vi "VFP.vi"() -> ()   [LabVIEW 2016]
uses:
  <vilib>/Utility/error.llb/DialogType.ctl
  states/InitializationStates.ctl
  states/DataAcqStates.ctl
  <vilib>/registry/registry.llb/Registry RtKey.ctl
  <vilib>/registry/registry.llb/Registry SAM.ctl
  <vilib>/Utility/error.llb/whitespace.ctl
  <vilib>/Analysis/baseanly.llb/Mean (DBL).vi
  <vilib>/registry/registry.llb/Read Registry Value Simple STR.vi
  Instance           5 11Saved   VFP .vi
  Instance          20 11Saved   VFP .vi
  Instance           6 11Saved   VFP .vi
  Instance          21 11Saved   VFP .vi
  Instance           8 11Saved   VFP .vi
  <vilib>/Analysis/NI_AALPro.lvlib
  <vilib>/Analysis/NI_AALBase.lvlib
panel:
  in  "Clear Graphs":bool
  out "Line of Best Fit":cluster{"type":sgl[], "Best Linear Fit":dbl[]}(graph)
  out "IV Data":cluster{"X":dbl[], "Y":dbl[]}[](graph)
  in  "Save on Start":bool
  out "Rough Resistance (MOhm)":dbl
  out "Done Time":dbl
  out "Current Time":dbl format="%_19f"
  in  "IV_Genfilname":bool
  in  "First Run IV":bool
  out "IV_start":dbl format="%_19f"
  out "Saving":bool
  out "?":path
  out "file or folder exists?":bool
  out "Target Resistance (adjusted Golovochenko)  (MOhm)":dbl
  out "Capillary Diameter (nm)":dbl
  in  "Bare Resistance \n(MOhm)":dbl
  out "Recording IV":bool
  in  "Start/Stop Saving":bool
  in  "Generate Filename":bool
  out "Control Amp Overload":bool caption="CA"
  out "Current Overload":bool caption="I"
  out "Voltage Overload":bool caption="V"
  in  "Legacy Save":bool
  out "Front Panel Window:Title 2":string="Gamry Instruments Virtual Front Panel"
  out "Log File Refnum 2":refnum<file>
  in  "Log File 2":path
  in  "Enable Section":bool
  in  "Desired Pore Size (nm)":dbl
  in  "Membrane Thickness \n(nm)":dbl
  in  "Sealed Resistance\n(MOhm)":dbl
  in  "Solution Conductance":dbl
  in  "Smoothing Parameter":i32=100
  out "Resistance (MOhm)":dbl
  out "Current(nA)":dbl
  in  "Select Graph":u16(ring) items=["V Vs. T, I vs. T", "I vs. V", "V vs. I"]
  out "Family":string
  out "Vf History":sgl[](array[numeric])
  out "Im History":sgl[](array[numeric])
  out "XY Graph Flipped?":bool
  in  "CA Speed":u16(ring)
  in  "I/E Stability":u16(ring)=2 items=["Fast", "Medium Fast", "Normal", "Slow"]
  in  "IchOffsetEnable":bool
  in  "VchOffsetEnable":bool
  in  "Ich Offset":sgl step=0.1 format="%^.3e"
  in  "Vch Offset":sgl step=0.1 format="%^.3e"
  in  "Ich Filter":u16(ring) items=["None", "200 kHz", "1 kHz", "5 Hz"]
  in  "Vch Filter":u16(ring) items=["None", "200 kHz", "1 kHz", "5 Hz"]
  in  "Ich Autorange":bool
  in  "Vch Autorange":bool
  in  "I/E Autorange":bool
  in  "I/E Range":u16(ring)=4 items=["60 pA", "600 pA", "6 nA", "60 nA", "600 nA", "6 µA", "60 µA", "600 µA", "6 mA", "60 mA", "600 mA"]
  in  "Ich Range":u16(ring) items=["30 mV", "300 mV", "3 V"]
  in  "Vch Range":u16(ring) items=["30 mV", "300 mV", "3 V", "12 V"]
  in  "Device":u16(ring) items=["REF600-17061"]
  in  "CtrlMode":u32(ring)=1 items=["Galvanostat", "Potentiostat", "ZRA"]
  in  "Continuous":bool=TRUE
  in  "Acq. Frequency":dbl=100.0 caption="Hz" min=0.001667 max=10000.0 step=1.0 format="%.3f"
  in  "Cycles":u32=1 min=1 step=1
  in  "Signal Type":u16(ring) items=["Take IV Curve"=9, "Sine Wave"=0, "Cosine Wave"=1, "Triangle"=2, "Square Wave"=3, "Sawtooth"=4, "Ramp"=5, "Single Point"=7, "From File"=8]
  in  "Filename":path
  in  "Phase Offset":dbl caption="Degrees" step=1.0 format="%.3f"
  in  "DC Offset":dbl caption="V" step=0.1 format="%^.3e"
  in  "Amplitude":dbl=0.1 caption="V" step=0.1 format="%^.3e"
  in  "Signal Frequency":dbl=1.0 caption="Hz" min=5e-05 max=300000.0 step=0.5 format="%.3f"
  in  "Final":dbl=0.5 caption="V" step=0.1 format="%^.3e"
  in  "Initial":dbl=-0.5 caption="V" step=0.1 format="%^.3e"
  in  "Duty Cycle":dbl=50.0 caption="Percent" min=0.0 max=100.0 step=0.1 format="%.3f"
  in  "Scan Rate":dbl=0.1 caption="V/s" step=0.01 format="%_3f"
  in  "Cell State":bool
  in  "Auto Cell Switch":bool=TRUE
  in  "Start/Stop":bool caption="Start"
  out "Confirm Exit?":bool
  out "?":sgl[][](graph)
  out "I vs. V":cluster{dbl, dbl}[](graph)
  out "SetCell":bool
  out "Cell Val Change NewVal":bool
  out "Version":string
  in  "[user-defined codes]":u32[](array[numeric])=[3758096430]
  in  "[user-defined descriptions]":string[](array[string])=["Device Not Authorized"]
  out "Taking Data":bool
  out "Front Panel Window:Title":string="Gamry Instruments Virtual Front Panel"
  in  "Log File":path
  out "Device Gone":bool
  out "Index of Device (Device Change)":i32
  out "milliseconds to wait":u32=150
  in  "Close":bool
  out "From File Refnum":refnum<file>
  out "Data Handlers":T1
  out "Log File Refnum":refnum<file>
  out "ForcePstatFunctionUpdate":bool
  out "File Data":string
  out "Device List Change Callback":refnum<k27>
  in  "Device List Change":bool
  out "Device Open":bool
  out "Section":string
  in  "GAMRYCOMLib.IGamrySignalArray":refnum<k7>
  in  "GAMRYCOMLib.IGamryDtaqIv":refnum<k7>
  in  "GAMRYCOMLib.IGamryPstat":refnum<k7>
  in  "GAMRYCOMLib.IGamryDeviceList":refnum<k7>
  out "DataDone Callback":refnum<k27>
  out "DataDone?":bool
  out "Dtaq Graph Callback":refnum<k27>
  in  "GAMRYCOMLib.IGamrySignal":refnum<k7>
  out "Signal":refnum<k7>
  out "Dtaq":refnum<k7>
  out "Pstat":refnum<k7>
  out "Device List":refnum<k7>
  out "First I/E Range":i32
  out "Section List":string[](array[string])=["PC5600-00002"]
  # "amoureux"
  # "Overloads"
  # "Save"
  # "Live View"
  # "1"
  # "2"
  # "displacing carbon atoms since 2018"
  # "Signal Generation"
  # "Nanopore Creator"
  # "Device Settings"
  # "Experiment Control"
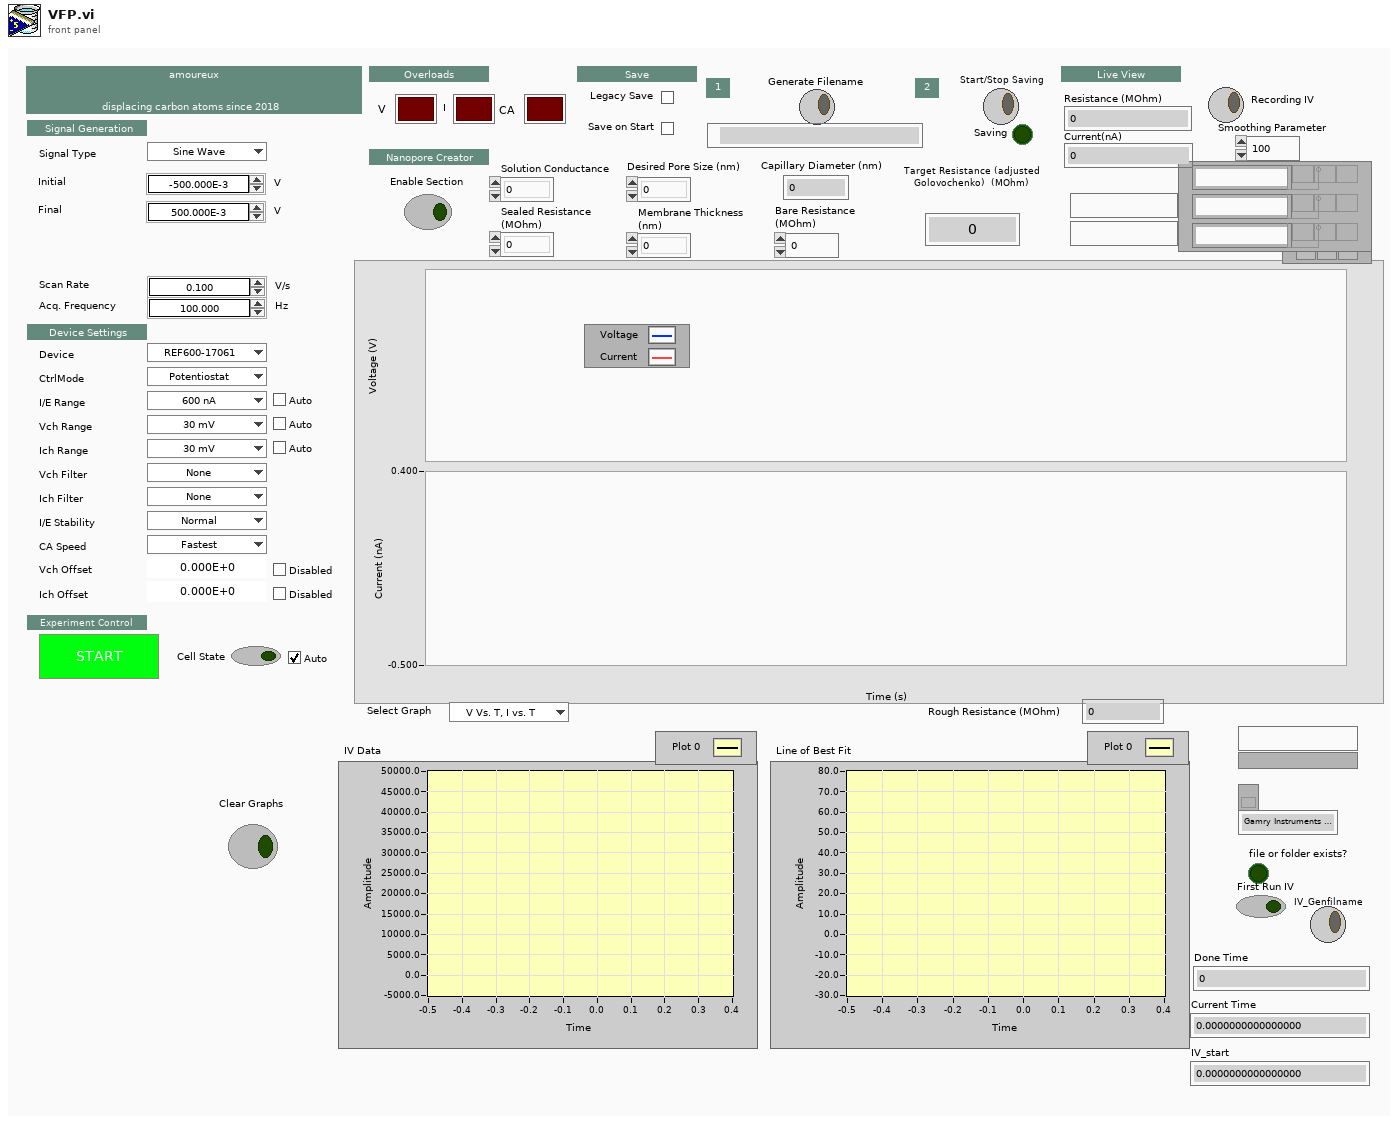
[diagram p1: front panel]
types:
  T1 = cluster{"Vs. T":refnum<vi>, "I vs. V":refnum<vi>, "Log File Refnum":refnum<vi>}
  T2 = typedef "InitializationStates.ctl" = enum16{"Initialize COM", "Load Device List", "Load Range Strings", "Setup Ranges", "Adjust Menu", "STOP"}
  T3 = typedef "DataAcqStates.ctl" = enum16{"Initialize", "Initialize Objects", "Generate Signal", "Data Acq Setup", "Acquire Data", "Cleanup", "STOP"}
  T4 = typedef "Registry SAM.ctl" = enum32{"KEY_QUERY_VALUE", "KEY_SET_VALUE", "KEY_CREATE_SUB_KEY", "KEY_ENUMERATE_SUB_KEYS", "KEY_NOTIFY", "KEY_CREATE_LINK", "KEY_READ", "KEY_WRITE", "KEY_ALL_ACCESS", "KEY_READ | KEY_WRITE"}
  T5 = typedef "Registry RtKey.ctl" = enum32{"HKEY_CLASSES_ROOT", "HKEY_CURRENT_USER", "HKEY_LOCAL_MACHINE", "HKEY_USERS", "HKEY_PERFORMANCE_DATA", "HKEY_CURRENT_CONFIG", "HKEY_DYN_DATA"}
  T6 = enum16{"open", "open or create", "create or replace", "create", "open (read only)"}
  T7 = cluster{"Ctrl Reference":refnum<vi>, "I vs. V":refnum<vi>, "Log File Refnum":refnum<vi>}
  T8 = cluster{"I/E Ranges":string[], "First I/E Range":i32, "VchRanges":string[], "IchRanges":string[], "AchRanges":string[], "VchFilters":string[], "IchFilters":string[], "AchFilters":string[], "Family":string, "CA Speeds":string[]}
  T9 = enum32{"existing file", "new file", "new or existing file", "existing dir", "new dir", "new or existing dir", "existing file (use LLBs)", "new file (use LLBs)", "new or existing file (use LLBs)", "new or existing file or directory (use LLBs)"}
  T10 = typedef "Registry refnum.ctl" = refnum<k1>
  T11 = typedef "whitespace.ctl" = u16
  T12 = cluster{"I Overload":bool, "CA Overload":bool, "V Overload":bool, "I ADC Railed":bool, "V ADC Railed":bool}
  T13 = enum32{"invalid app kind", "Development System", "Run Time System", "Student Edition", "Embedded LabVIEW", "Evaluation", "Custom"}
  T14 = typedef "DialogType.ctl" = u16
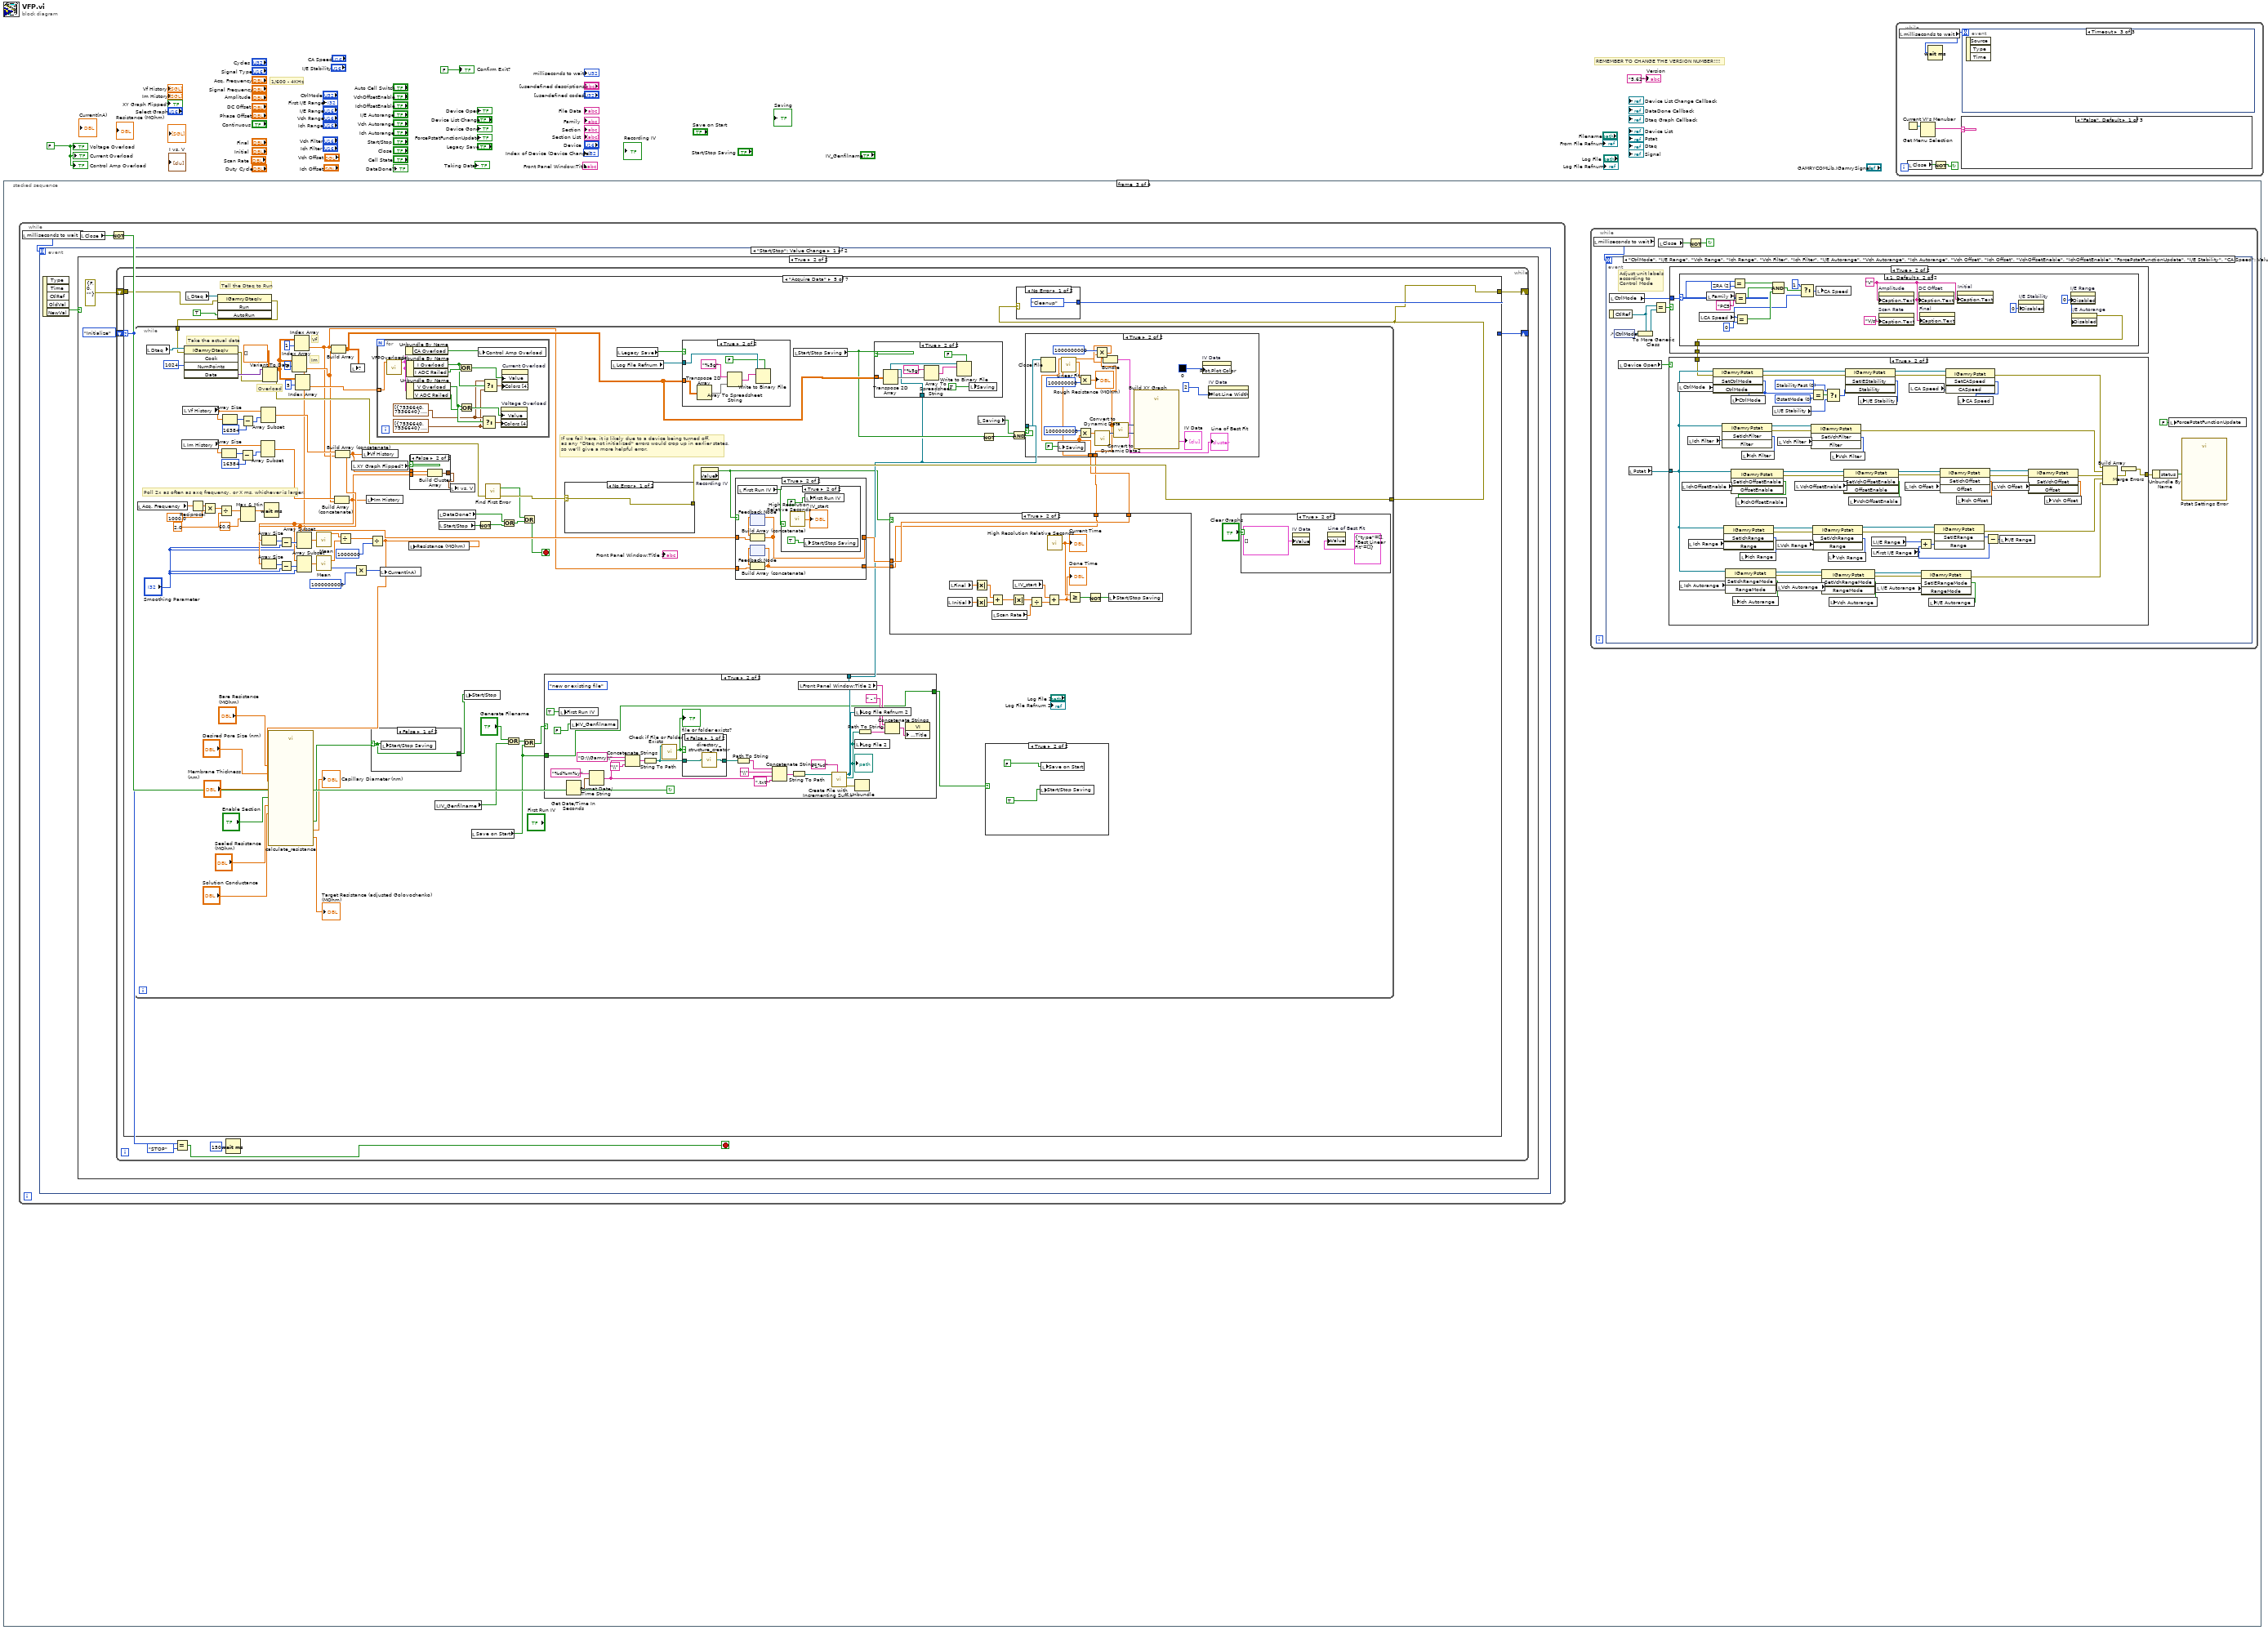
[diagram p0: block diagram]
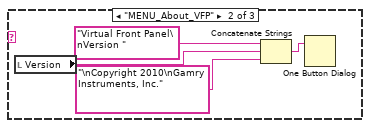
[diagram p2: hidden frame]
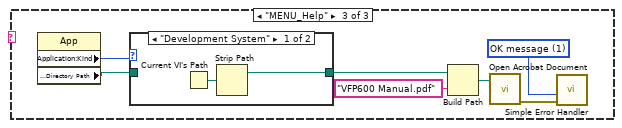
[diagram p3: hidden frame]
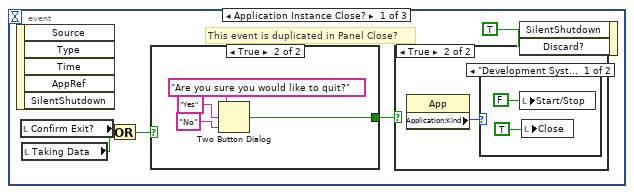
[diagram p5: hidden frame]
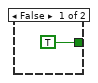
[diagram p6: hidden frame]
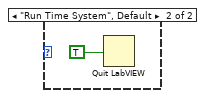
[diagram p8: hidden frame]
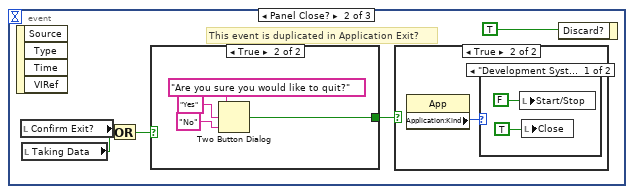
[diagram p9: hidden frame]
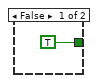
[diagram p10: hidden frame]
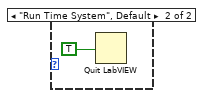
[diagram p12: hidden frame]
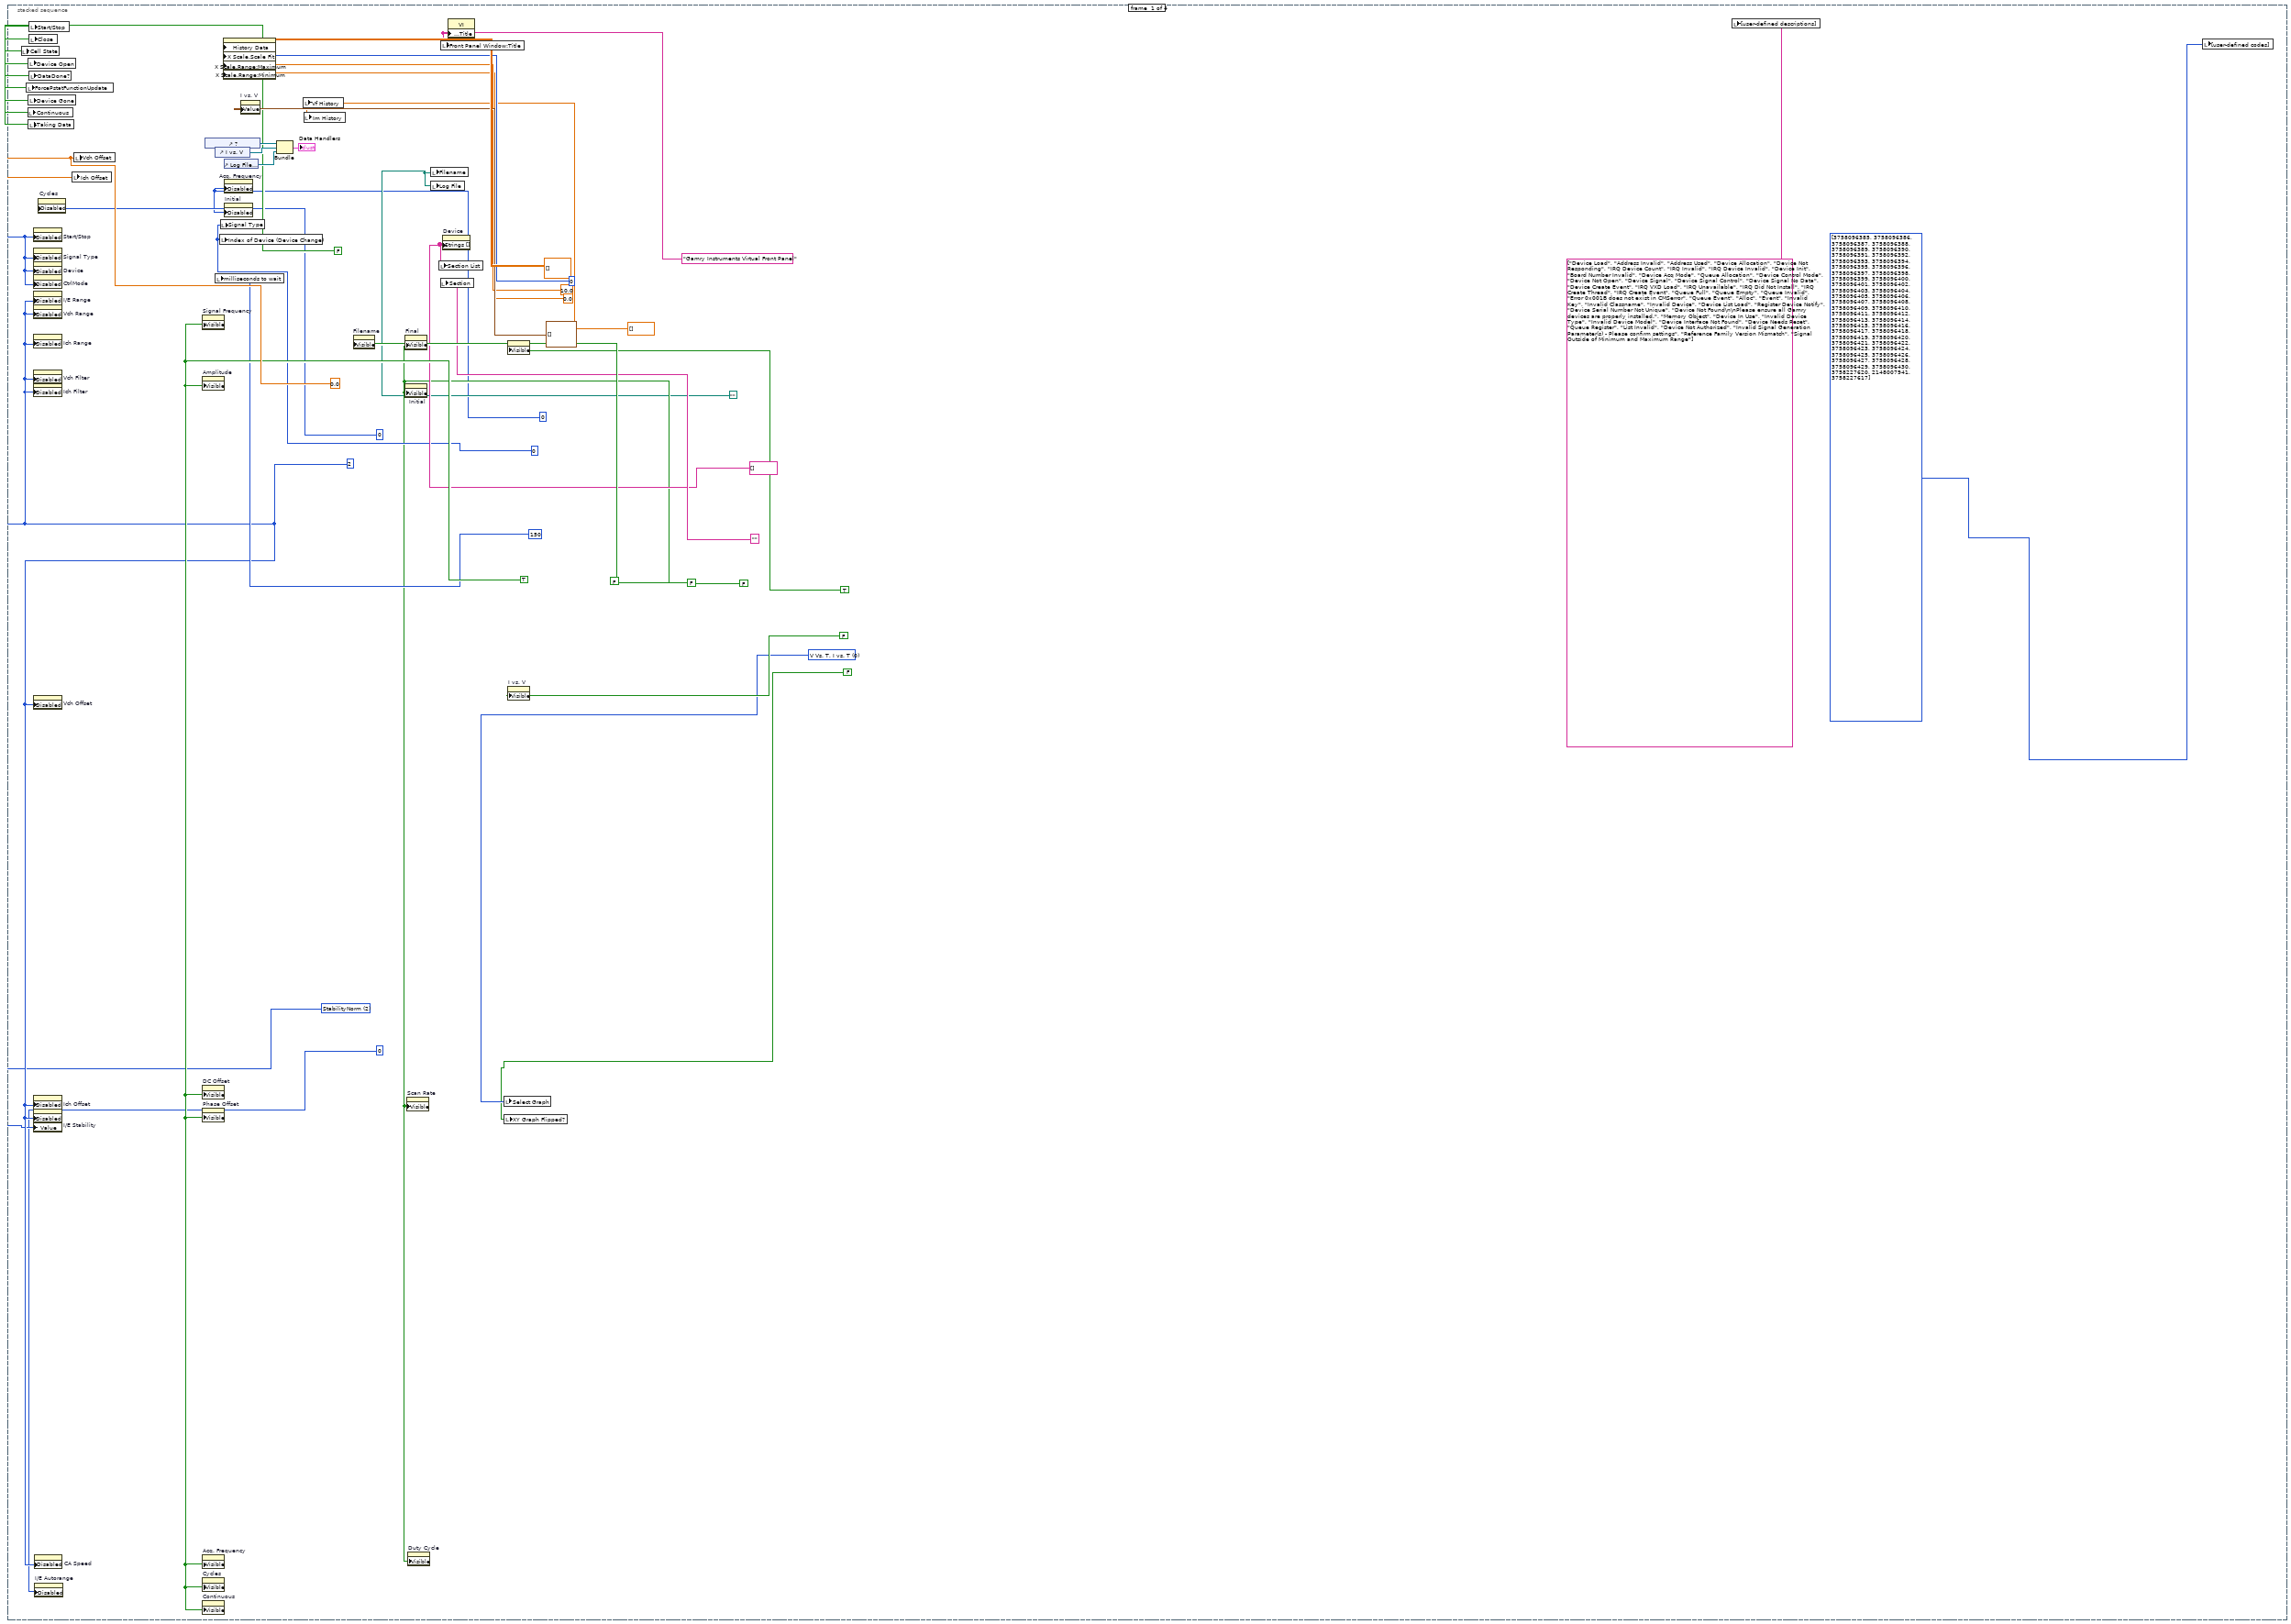
[diagram p13: hidden frame]
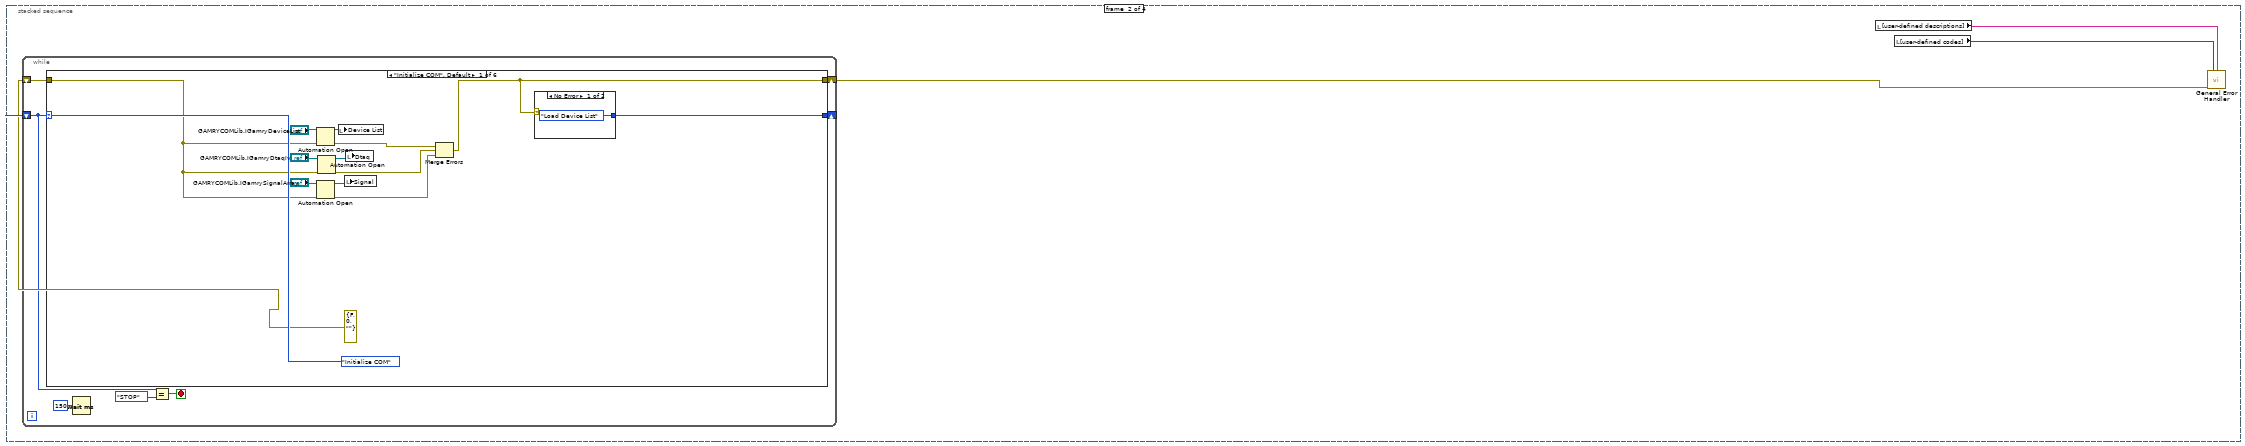
[diagram p14: hidden frame]
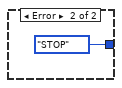
[diagram p15: hidden frame]
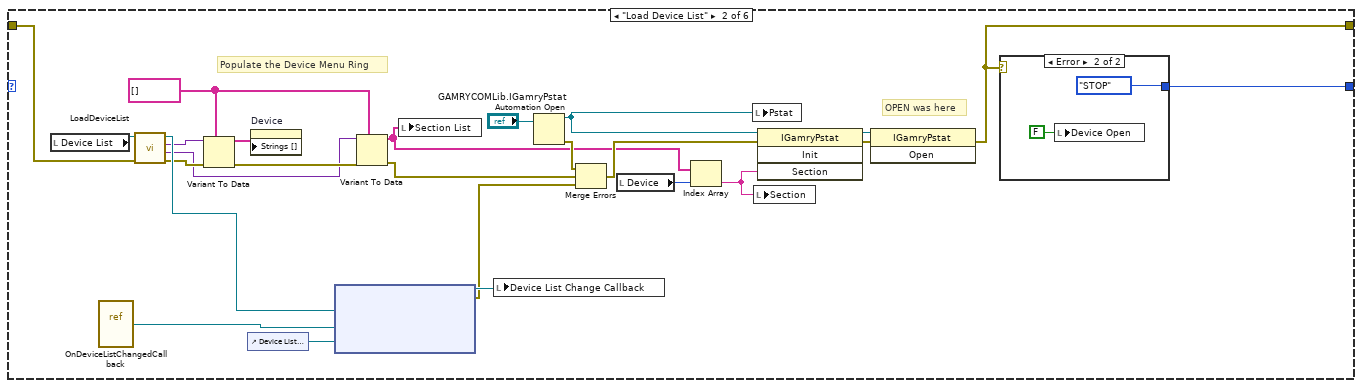
[diagram p16: hidden frame]
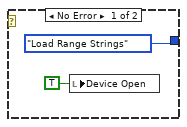
[diagram p17: hidden frame]
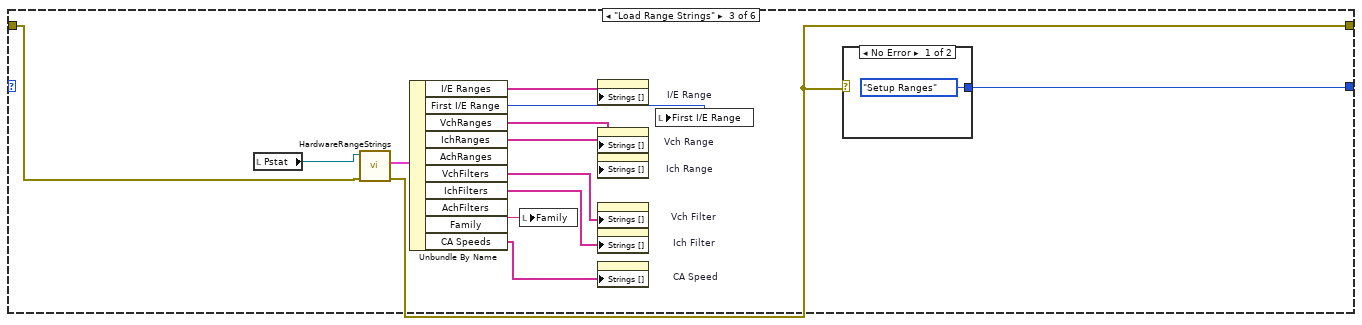
[diagram p18: hidden frame]
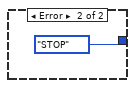
[diagram p19: hidden frame]
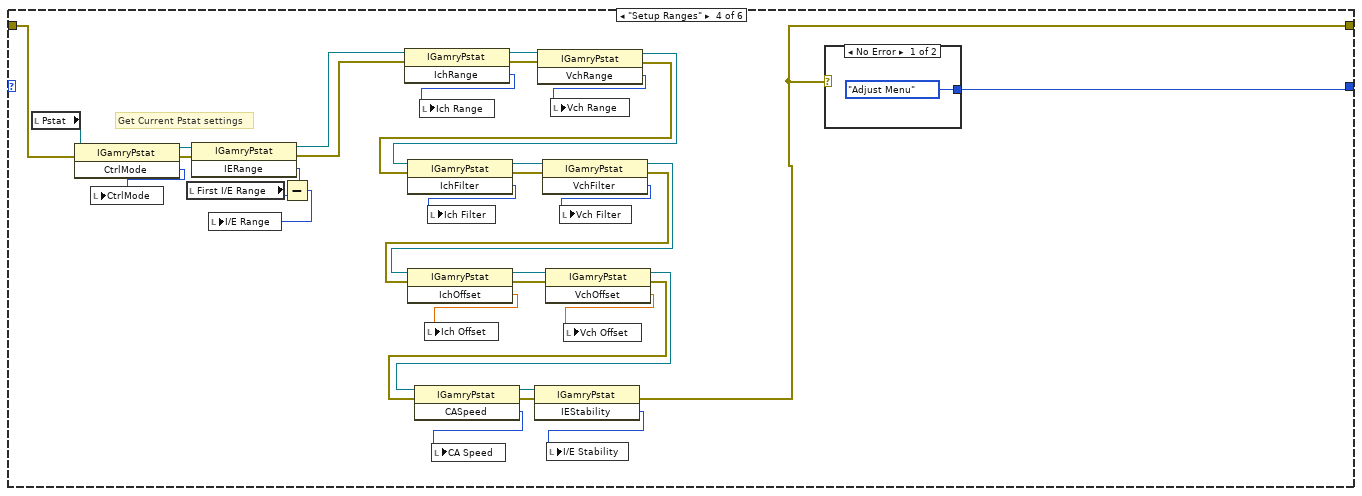
[diagram p20: hidden frame]
diagram:
  w1 = FALSE
  # "REMEMBER TO CHANGE THE VERSION NUMBER!!!!"
  # "1/600 - 4KHz"
  n1 = stacked-sequence {
    frame #0 {
      w5 = sgl[] [] ("Vf History")
      w7 = u16 0 items=["V Vs. T, I vs. T", "I vs. V", "V vs. I"] ("Select Graph")
      w12 = path ""
      w13 = 2 items=["StabilityFast", "StabilityMedFast", "StabilityNorm", "StabilitySlow"] ("Stability")
      w20 = "Gamry Instruments Virtual Front Panel" ("Front Panel Window:Title")
      w15 = FALSE ("Visible")
      w8 = u8 0 ("Disabled")
      w14 = u8 2 ("Disabled")
      (unwired) FALSE ("Visible")
      w30 = TRUE ("Visible")
      w34 = sgl 0.0 ("Vch Offset")
      w19 = FALSE ("I/E Autorange 2")
      w24 = u32 0 ("Zero")
      w25 = string[] [] ("Strings []")
      n2 = local write "Cell State"(w19) -> ()
      n3 = local write "ForcePstatFunctionUpdate"(w19) -> ()
      n4 = local write "Continuous"(w19) -> ()
      n5 = local write "Device Open"(w19) -> ()
      n6 = local write "Device Gone"(w19) -> ()
      n7 = local write "Taking Data"(w19) -> ()
      n8 = local write "DataDone?"(w19) -> ()
      n9 = local write "Start/Stop"(w19) -> ()
      n10 = local write "Close"(w19) -> ()
      n11 = property on="Start/Stop" class="Bool (strict)"("Disabled"=w14) -> ()  [unwired: 2 in, 2 out]
      n12 = property on="Signal Type" class="Ring (strict)"("Disabled"=w14) -> ()  [unwired: 2 in, 2 out]
      n13 = property on="Device" class="Ring (strict)"("Disabled"=w14) -> ()  [unwired: 2 in, 2 out]
      n14 = property on="CtrlMode" class="Ring (strict)"("Disabled"=w14) -> ()  [unwired: 2 in, 2 out]
      n15 = property on="I/E Range" class="Ring (strict)"("Disabled"=w14) -> ()  [unwired: 2 in, 2 out]
      n16 = property on="Vch Range" class="Ring (strict)"("Disabled"=w14) -> ()  [unwired: 2 in, 2 out]
      n17 = property on="Ich Range" class="Ring (strict)"("Disabled"=w14) -> ()  [unwired: 2 in, 2 out]
      n18 = property on="Vch Filter" class="Ring (strict)"("Disabled"=w14) -> ()  [unwired: 2 in, 2 out]
      n19 = property on="Ich Filter" class="Ring (strict)"("Disabled"=w14) -> ()  [unwired: 2 in, 2 out]
      n20 = property on="Vch Offset" class="DigNum (strict)"("Disabled"=w14) -> ()  [unwired: 2 in, 2 out]
      n21 = property on="Ich Offset" class="DigNum (strict)"("Disabled"=w14) -> ()  [unwired: 2 in, 2 out]
      n22 = property on="I/E Stability" class="Ring (strict)"("Disabled"=w14, "Value"=w13) -> ()  [unwired: 2 in, 2 out]
      n23 = property on="CA Speed" class="Ring (strict)"("Disabled"=w14) -> ()  [unwired: 2 in, 2 out]
      n24 = property on="I/E Autorange" class="Bool (strict)"("Disabled"=u8 0) -> ()  [unwired: 2 in, 2 out]
      n25 = property on="Cycles" class="DigNum (strict)"("Disabled"=0) -> ()  [unwired: 2 in, 2 out]
      n26 = local write "Ich Offset"(w34) -> ()
      n27 = local write "Vch Offset"(w34) -> ()
      n28 = property on="Signal Frequency" class="DigNum (strict)"("Visible"=w30) -> ()  [unwired: 2 in, 2 out]
      n29 = property on="Amplitude" class="DigNum (strict)"("Visible"=w30) -> ()  [unwired: 2 in, 2 out]
      n30 = property on="DC Offset" class="DigNum (strict)"("Visible"=w30) -> ()  [unwired: 2 in, 2 out]
      n31 = property on="Phase Offset" class="DigNum (strict)"("Visible"=w30) -> ()  [unwired: 2 in, 2 out]
      n32 = property on="Acq. Frequency" class="DigNum (strict)"("Visible"=w30) -> ()  [unwired: 2 in, 2 out]
      n33 = property on="Cycles" class="DigNum (strict)"("Visible"=w30) -> ()  [unwired: 2 in, 2 out]
      n34 = property on="Continuous" class="Bool (strict)"("Visible"=w30) -> ()  [unwired: 2 in, 2 out]
      n35 = control-ref of="?"() -> (w33:refnum<vi>)
      n36 = control-ref of="I vs. V"() -> (w32:refnum<vi>)
      n37 = local write "milliseconds to wait"(u32 150 ("milliseconds to wait")) -> ()
      n38 = local write "Index of Device (Device Change)"(w24) -> ()
      n39 = local write "Signal Type"(w24) -> ()
      n40 = property class="WFChart (strict)"("History Data"=sgl[][] [], "X Scale.Scale Fit"=u8 0, "X Scale.Range:Maximum"=10.0, "X Scale.Range:Minimum"=0.0) -> ()  [unwired: 2 in, 2 out]
      n41 = control-ref of="Log File Refnum"() -> (w28:refnum<vi>)
      n42 = property on="Acq. Frequency" class="DigNum (strict)"("Disabled"=w8) -> ()  [unwired: 2 in, 2 out]
      n43 = property on="Initial" class="DigNum (strict)"("Disabled"=w8) -> ()  [unwired: 2 in, 2 out]
      n44 = property on="I vs. V" class="XYGraph (strict)"("Value"=cluster{dbl, dbl}[] [] ("I vs. V")) -> ()  [unwired: 2 in, 2 out]
      n45 = Bundle("Ctrl Reference"=w33, "I vs. V"=w32, "Log File Refnum"=w28) -> (→"Data Handlers":T7)  [unwired: 1 in]
      n46 = local write "Vf History"(w5) -> ()
      n47 = local write "Im History"(w5) -> ()
      n48 = property on="Filename" class="Path"("Visible"=FALSE) -> ()  [unwired: 2 in, 2 out]
      n49 = property on="Final" class="DigNum (strict)"("Visible"=w15) -> ()  [unwired: 2 in, 2 out]
      n50 = property on="Initial" class="DigNum (strict)"("Visible"=w15) -> ()  [unwired: 2 in, 2 out]
      n51 = property on="Scan Rate" class="DigNum (strict)"("Visible"=w15) -> ()  [unwired: 2 in, 2 out]
      n52 = property on="Duty Cycle" class="DigNum (strict)"("Visible"=w15) -> ()  [unwired: 2 in, 2 out]
      n53 = local write "Filename"(w12) -> ()
      n54 = local write "Log File"(w12) -> ()
      n55 = local write "Section List"(w25) -> ()
      n56 = local write "Section"("" ("Section")) -> ()
      n57 = local write "Front Panel Window:Title"(w20) -> ()
      n58 = property on="Device" class="Ring (strict)"("Strings []"=w25) -> ()  [unwired: 2 in, 2 out]
      n59 = property class="VI"("Front Panel Window:Title"=w20) -> ()  [unwired: 2 in, 2 out]
      n60 = local write "Select Graph"(w7) -> ()
      n61 = local write "XY Graph Flipped?"(FALSE ("XY Graph Flipped?")) -> ()
      n62 = property class="WFChart (strict)"("Visible"=TRUE) -> ()  [unwired: 2 in, 2 out]
      n63 = property on="I vs. V" class="XYGraph (strict)"("Visible"=FALSE) -> ()  [unwired: 2 in, 2 out]
      n64 = local write "[user-defined descriptions]"(string[] ["Device Load", "Address Invalid", "Address Used", "Device Allocation", "Device Not Responding", "IRQ Device Count", "IRQ Invalid", "IRQ Device Invalid", "Device Init", "Board Number Invalid", "Device Acq Mode", "Queue Allocation", "Device Control Mode", "Device Not Open", "Device Signal", "Device Signal Control", "Device Signal No Data", "Device Create Event", "IRQ VXD Load", "IRQ Unavailable", "IRQ Did Not Install", "IRQ Create Thread", "IRQ Create Event", "Queue Full", "Queue Empty", "Queue Invalid", "Error 0x001B does not exist in CMSerror", "Queue Event", "Alloc", "Event", "Invalid Key", "Invalid Classname", "Invalid Device", "Device List Load", "Register Device Notify", "Device Serial Number Not Unique", "Device Not Found\n\nPlease ensure all Gamry devices are properly installed.", "Memory Object", "Device In Use", "Invalid Device Type", "Invalid Device Model", "Device Interface Not Found", "Device Needs Reset", "Queue Register", "List Invalid", "Device Not Authorized", "Invalid Signal Generation Parameter(s) - Please confirm settings", "Reference Family Version Mismatch", "Signal Outside of Minimum and Maximum Range"] ("[user-defined descriptions]")) -> ()
      n65 = local write "[user-defined codes]"(u32[] [3758096385, 3758096386, 3758096387, 3758096388, 3758096389, 3758096390, 3758096391, 3758096392, 3758096393, 3758096394, 3758096395, 3758096396, 3758096397, 3758096398, 3758096399, 3758096400, 3758096401, 3758096402, 3758096403, 3758096404, 3758096405, 3758096406, 3758096407, 3758096408, 3758096409, 3758096410, 3758096411, 3758096412, 3758096413, 3758096414, 3758096415, 3758096416, 3758096417, 3758096418, 3758096419, 3758096420, 3758096421, 3758096422, 3758096423, 3758096424, 3758096425, 3758096426, 3758096427, 3758096428, 3758096429, 3758096430, 3758227620, 2148007941, 3758227617] ("[user-defined codes]")) -> ()
    }
    frame #1 {
      n66 = while {
        shift-right: [w41] -> _
        shift-left: InitializationStates."Initialize COM" ("Initialization States") -> [w47]
        shift-right: [w43] -> w36
        shift-left: errorcluster {"status"=FALSE, "code"=0, "source"=""} ("error out") -> [w42]
        stop <- w45 stop-if-true
        n67 = case shown="\"Initialize COM\", Default" w47 {
          tunnel: [w49 w62 w91 w106 w142 w161] -> w43
          tunnel: w42 -> [w50 w67 w93 w133 w143 w161]
          tunnel: [w48 w65 w97 w132 w151 InitializationStates."STOP" ("Initialization States")] -> w41
          frame "Initialize COM", Default {
            n68 = Automation Open(error in (no error)=w50, Automation Refnum="GAMRYCOMLib.IGamryDeviceList") -> (Automation Refnum=w59:refnum<k7>, error out=w56:errorcluster)  [unwired: 2 in]
            n69 = Automation Open(error in (no error)=w50, Automation Refnum="GAMRYCOMLib.IGamrySignalArray") -> (Automation Refnum=w52:refnum<k7>, error out=w58:errorcluster)  [unwired: 2 in]
            n70 = Automation Open(error in (no error)=w50, Automation Refnum="GAMRYCOMLib.IGamryDtaqIv") -> (Automation Refnum=w51:refnum<k7>, error out=w57:errorcluster)  [unwired: 2 in]
            n71 = local write "Device List"(w59) -> ()
            n72 = local write "Signal"(w52) -> ()
            n73 = local write "Dtaq"(w51) -> ()
            n74 = Merge Errors(w56, w57, w58) -> (w49:errorcluster)
            n75 = case shown="No Error" w49 {
              tunnel: [InitializationStates."Load Device List" ("Initialization States") InitializationStates."STOP" ("Initialization States")] -> w48
              frame No Error {
              }
              frame Error {
              }
            }
          }
          frame "Load Device List" {
            w69 = string[] []
            # "OPEN was here"
            # "Populate the Device Menu Ring"
            n76 = local read "Device List"() -> (w86:refnum<k7>)
            n77 = vi-ref "OnDeviceListChangedCallback.vi"() -> ("vi reference"=w75:refnum<vi>)
            n78 = call "LoadDeviceList.vi"("Error In"=w67, "GAMRYCOMLib.IGamryDeviceList In"=w86) -> ("Error Out"=w82:errorcluster, "EnumSections"=w81:variant, "EnumLabels"=w80:variant, "GAMRYCOMLib.IGamryDeviceList Out"=w85:refnum<k7>)  [unwired: 4 in]
            n79 = Variant To Data(error in=w82, type=w69, Variant=w80) -> (data=w68:string[], error out=w84:errorcluster)
            n80 = control-ref of="Device List Change"() -> (w74:refnum<vi>)
            n81 = property on="Device" class="Ring (strict)"("Strings []"=w68) -> ()  [unwired: 2 in, 2 out]
            n82 = node(w85, w75, w74) -> (w76:refnum<k27>, w66:errorcluster)  [unwired: 2 in]
            n83 = Variant To Data(error in=w84, type=w69, Variant=w81) -> (data=w77:string[], error out=w83:errorcluster)
            n84 = local write "Section List"(w77) -> ()
            n85 = local write "Device List Change Callback"(w76) -> ()
            n86 = Automation Open(Automation Refnum="GAMRYCOMLib.IGamryPstat") -> (Automation Refnum=w73:refnum<k7>, error out=w78:errorcluster)  [unwired: 3 in]
            n87 = Merge Errors(w78, w83, w66) -> (w79:errorcluster)
            n88 = local read "Device"() -> (w71:u16)
            n89 = Index Array(array=w77, index=w71) -> (element=w72:string)
            n90 = local write "Pstat"(w73) -> ()
            n91 = local write "Section"(w72) -> ()
            n92 = invoke class="IGamryPstat" method="Init"(reference=w73, error in=w79, "Section"=w72) -> (reference out=w63:refnum<k7>, error out=w64:errorcluster)  [unwired: 1 in, 2 out]
            n93 = invoke class="IGamryPstat" method="Open"(reference=w63, error in=w64) -> (error out=w62:errorcluster)  [unwired: 1 in, 2 out]
            n94 = case shown="Error" w62 {
              tunnel: [InitializationStates."Load Range Strings" ("Initialization States") InitializationStates."STOP" ("Initialization States")] -> w65
              frame No Error {
                n95 = local write "Device Open"(TRUE ("Device Open")) -> ()
              }
              frame Error {
                n96 = local write "Device Open"(FALSE ("Device Open")) -> ()
              }
            }
          }
          frame "Load Range Strings" {
            n97 = local read "Pstat"() -> (w94:refnum<k7>)
            n98 = call "HardwareRangeStrings.vi"("error in (no error)"=w93, "Pstat IN"=w94) -> ("error out"=w91:errorcluster, "Hardware Strings"=w92:T8)  [unwired: 7 in, 1 out]
            n99 = Unbundle By Name(w92) -> ("I/E Ranges"=w101:string[], "First I/E Range"=w98:i32, "VchRanges"=w99:string[], "IchRanges"=w100:string[], "VchFilters"=w102:string[], "IchFilters"=w103:string[], "Family"=w95:string, "CA Speeds"=w96:string[])  [unwired: 2 out]
            n100 = local write "Family"(w95) -> ()
            n101 = property on="I/E Range" class="Ring (strict)"("Strings []"=w101) -> ()  [unwired: 2 in, 2 out]
            n102 = property on="Vch Range" class="Ring (strict)"("Strings []"=w99) -> ()  [unwired: 2 in, 2 out]
            n103 = property on="Ich Range" class="Ring (strict)"("Strings []"=w100) -> ()  [unwired: 2 in, 2 out]
            n104 = property on="Vch Filter" class="Ring (strict)"("Strings []"=w102) -> ()  [unwired: 2 in, 2 out]
            n105 = property on="Ich Filter" class="Ring (strict)"("Strings []"=w103) -> ()  [unwired: 2 in, 2 out]
            n106 = property on="CA Speed" class="Ring (strict)"("Strings []"=w96) -> ()  [unwired: 2 in, 2 out]
            n107 = local write "First I/E Range"(w98) -> ()
            n108 = case shown="No Error" w91 {
              tunnel: [InitializationStates."Setup Ranges" ("Initialization States") InitializationStates."STOP" ("Initialization States")] -> w97
              frame No Error {
              }
              frame Error {
              }
            }
          }
          frame "Setup Ranges" {
            # "Get Current Pstat settings"
            n109 = local read "Pstat"() -> (w134:refnum<k7>)
            n110 = invoke class="IGamryPstat" method="CtrlMode"(reference=w134, error in=w133) -> (reference out=w138:refnum<k7>, error out=w139:errorcluster, "CtrlMode"=w136:i32)  [unwired: 1 in]
            n111 = local write "CtrlMode"(w136) -> ()
            n112 = local read "First I/E Range"() -> (w131:i32)
            n113 = invoke class="IGamryPstat" method="IERange"(reference=w138, error in=w139) -> (reference out=w108:refnum<k7>, error out=w107:errorcluster, "IERange"=w135:i32)  [unwired: 1 in]
            n114 = Subtract(x=w135, y=w131) -> (x-y=w137:i32)
            n115 = local write "I/E Range"(w137) -> ()
            n116 = invoke class="IGamryPstat" method="IchRange"(reference=w108, error in=w107) -> (reference out=w113:refnum<k7>, error out=w112:errorcluster, "IchRange"=w110:i32)  [unwired: 1 in]
            n117 = local write "Ich Range"(w110) -> ()
            n118 = invoke class="IGamryPstat" method="VchRange"(reference=w113, error in=w112) -> (reference out=w126:refnum<k7>, error out=w109:errorcluster, "VchRange"=w111:i32)  [unwired: 1 in]
            n119 = invoke class="IGamryPstat" method="IchFilter"(reference=w126, error in=w109) -> (reference out=w121:refnum<k7>, error out=w120:errorcluster, "IchFilter"=w122:i32)  [unwired: 1 in]
            n120 = local write "Ich Filter"(w122) -> ()
            n121 = invoke class="IGamryPstat" method="VchFilter"(reference=w121, error in=w120) -> (reference out=w128:refnum<k7>, error out=w127:errorcluster, "VchFilter"=w123:i32)  [unwired: 1 in]
            n122 = invoke class="IGamryPstat" method="IchOffset"(reference=w128, error in=w127) -> (reference out=w118:refnum<k7>, error out=w119:errorcluster, "IchOffset"=w124:sgl)  [unwired: 1 in]
            n123 = local write "Ich Offset"(w124) -> ()
            n124 = invoke class="IGamryPstat" method="VchOffset"(reference=w118, error in=w119) -> (reference out=w130:refnum<k7>, error out=w129:errorcluster, "VchOffset"=w125:sgl)  [unwired: 1 in]
            n125 = invoke class="IGamryPstat" method="CASpeed"(reference=w130, error in=w129) -> (reference out=w114:refnum<k7>, error out=w115:errorcluster, "CASpeed"=w117:i32)  [unwired: 1 in]
            n126 = local write "CA Speed"(w117) -> ()
            n127 = invoke class="IGamryPstat" method="IEStability"(reference=w114, error in=w115) -> (error out=w106:errorcluster, "IEStability"=w116:i32)  [unwired: 1 in, 1 out]
            n128 = local write "I/E Stability"(w116) -> ()
            n129 = local write "Vch Range"(w111) -> ()
            n130 = local write "Vch Filter"(w123) -> ()
            n131 = local write "Vch Offset"(w125) -> ()
            n132 = case shown="No Error" w106 {
              tunnel: [InitializationStates."Adjust Menu" ("Initialization States") InitializationStates."STOP" ("Initialization States")] -> w132
              frame No Error {
              }
              frame Error {
              }
            }
          }
          frame "Adjust Menu" {
            n133 = local read "CtrlMode"() -> (w150:u32)
            n134 = case shown="0" w150 {
              tunnel: ["V" ("Caption.Text") "A" ("Caption.Text")] -> w149
              tunnel: ["V/s" ("Caption.Text") "A/s" ("Caption.Text")] -> w148
              frame 1, Default {
              }
              frame 0 {
              }
            }
            n135 = property on="Amplitude" class="DigNum (strict)"(error in=w143, "Caption.Text"=w149) -> (error out=w147:errorcluster)  [unwired: 1 in, 1 out]
            n136 = property on="DC Offset" class="DigNum (strict)"(error in=w147, "Caption.Text"=w149) -> (error out=w146:errorcluster)  [unwired: 1 in, 1 out]
            n137 = property on="Initial" class="DigNum (strict)"(error in=w146, "Caption.Text"=w149) -> (error out=w145:errorcluster)  [unwired: 1 in, 1 out]
            n138 = property on="Final" class="DigNum (strict)"(error in=w145, "Caption.Text"=w149) -> (error out=w144:errorcluster)  [unwired: 1 in, 1 out]
            n139 = property on="Scan Rate" class="DigNum (strict)"(error in=w144, "Caption.Text"=w148) -> (error out=w142:errorcluster)  [unwired: 1 in, 1 out]
            n140 = case shown="Error" w142 {
              tunnel: [InitializationStates."STOP" ("Initialization States") InitializationStates."STOP" ("Initialization States")] -> w151
              frame No Error {
                w156 = u8 0 ("Disabled")
                # "Enable appropriate menu stuff"
                n141 = property on="Start/Stop" class="Bool (strict)"("Disabled"=w156) -> ()  [unwired: 2 in, 2 out]
                n142 = property on="Device" class="Ring (strict)"("Disabled"=w156) -> ()  [unwired: 2 in, 2 out]
                n143 = property on="CtrlMode" class="Ring (strict)"("Disabled"=w156) -> ()  [unwired: 2 in, 2 out]
                n144 = property on="Signal Type" class="Ring (strict)"("Disabled"=w156) -> ()  [unwired: 2 in, 2 out]
                n145 = property on="I/E Range" class="Ring (strict)"("Disabled"=w156) -> ()  [unwired: 2 in, 2 out]
                n146 = property on="Vch Range" class="Ring (strict)"("Disabled"=w156) -> ()  [unwired: 2 in, 2 out]
                n147 = property on="Ich Range" class="Ring (strict)"("Disabled"=w156) -> ()  [unwired: 2 in, 2 out]
                n148 = property on="Vch Filter" class="Ring (strict)"("Disabled"=w156) -> ()  [unwired: 2 in, 2 out]
                n149 = property on="Ich Filter" class="Ring (strict)"("Disabled"=w156) -> ()  [unwired: 2 in, 2 out]
                n150 = property on="Vch Offset" class="DigNum (strict)"("Disabled"=w156) -> ()  [unwired: 2 in, 2 out]
                n151 = property on="Ich Offset" class="DigNum (strict)"("Disabled"=w156) -> ()  [unwired: 2 in, 2 out]
                n152 = property on="I/E Stability" class="Ring (strict)"("Disabled"=w156) -> ()  [unwired: 2 in, 2 out]
                n153 = property on="CA Speed" class="Ring (strict)"("Disabled"=w156) -> ()  [unwired: 2 in, 2 out]
              }
              frame Error {
                w160 = u16 0 items=[""] ("Device")
                w158 = u8 2 ("Disabled")
                # "Disable appropriate menu stuff"
                n154 = property on="Start/Stop" class="Bool (strict)"("Disabled"=w158) -> ()  [unwired: 2 in, 2 out]
                n155 = property on="CtrlMode" class="Ring (strict)"("Disabled"=w158) -> ()  [unwired: 2 in, 2 out]
                n156 = property on="Device" class="Ring (strict)"("Disabled"=w158, "Value"=w160) -> ()  [unwired: 2 in, 2 out]
                n157 = property on="I/E Range" class="Ring (strict)"("Disabled"=w158, "Value"=w160) -> ()  [unwired: 2 in, 2 out]
                n158 = property on="Vch Range" class="Ring (strict)"("Disabled"=w158, "Value"=w160) -> ()  [unwired: 2 in, 2 out]
                n159 = property on="Ich Range" class="Ring (strict)"("Disabled"=w158, "Value"=w160) -> ()  [unwired: 2 in, 2 out]
                n160 = property on="Vch Filter" class="Ring (strict)"("Disabled"=w158, "Value"=w160) -> ()  [unwired: 2 in, 2 out]
                n161 = property on="Ich Filter" class="Ring (strict)"("Disabled"=w158, "Value"=w160) -> ()  [unwired: 2 in, 2 out]
                n162 = property on="Vch Offset" class="DigNum (strict)"("Disabled"=w158) -> ()  [unwired: 2 in, 2 out]
                n163 = property on="Ich Offset" class="DigNum (strict)"("Disabled"=w158) -> ()  [unwired: 2 in, 2 out]
                n164 = property on="I/E Stability" class="Ring (strict)"("Disabled"=w158) -> ()  [unwired: 2 in, 2 out]
                n165 = property on="CA Speed" class="Ring (strict)"("Disabled"=w158) -> ()  [unwired: 2 in, 2 out]
              }
            }
          }
          frame "STOP" {
          }
        }
        n166 = Wait (ms)(milliseconds to wait=u32 150) -> ()  [unwired: 1 out]
        n167 = Equal?(x=w47, y=InitializationStates."STOP" ("Initialization States")) -> (x = y?=w45:bool)
      }
      n168 = local read "[user-defined descriptions]"() -> (w40:string[])
      n169 = local read "[user-defined codes]"() -> (w39:u32[])
      n170 = call <vilib>:"General Error Handler.vi"("[user-defined codes]"=w39, "[user-defined descriptions]"=w40, "error in (no error)"=w36) -> ()  [unwired: 8 in, 5 out]
    }
    frame #2 {
      n171 = while {
        stop <- w655 continue-if-true
        n172 = local read "milliseconds to wait"() -> (w654:u32)
        n173 = event shown="[0] \"Start/Stop\": Value Change" {
          selector: _ -> [_ _]
          dyn-events: _ -> [_ _]
          timeout: w654 -> [_ _]
          event "Start/Stop": Value Change {
            n174 = event-data() -> ("NewVal"=w657:bool)  [unwired: 1 in, 4 out]
            n175 = case shown="True" w657 {
              frame False {
              }
              frame True {
                n176 = while {
                  shift-right: [w662] -> _
                  shift-left: DataAcqStates."Initialize" ("Data Acq States") -> [w665]
                  shift-right: [w660] -> _
                  shift-left: errorcluster {"status"=FALSE, "code"=0, "source"=""} ("error in (no error)") -> [w661]
                  stop <- w666 stop-if-true
                  n177 = case shown="\"Acquire Data\"" w665 {
                    tunnel: [DataAcqStates."Initialize Objects" ("Data Acq States") w732 w747 w937 w955 w1174 DataAcqStates."STOP" ("Data Acq States")] -> w662
                    tunnel: w661 -> [w671 w712 w748 w940 w956 w1176 w1213]
                    tunnel: [w671 w722 w742 w938 w954 w1173 w1204] -> w660
                    frame "Initialize", Default {
                      w667 = u8 2 ("Disabled")
                      w669 = path "" ("Log File")
                      w670 = sgl[] [] ("Vf History")
                      w668 = FALSE
                      # "Disable appropriate menu items"
                      # "Initalize Chart and Lists"
                      n178 = local read "Continuous"() -> (w677:bool)
                      n179 = property on="CtrlMode" class="Ring (strict)"("Disabled"=w667) -> ()  [unwired: 2 in, 2 out]
                      n180 = property on="Legacy Save" class="Bool (strict)"("Disabled"=w667) -> ()  [unwired: 2 in, 2 out]
                      n181 = property on="Device" class="Ring (strict)"("Disabled"=w667) -> ()  [unwired: 2 in, 2 out]
                      n182 = property on="Acq. Frequency" class="DigNum (strict)"("Disabled"=w667) -> ()  [unwired: 2 in, 2 out]
                      n183 = Select(t=2, s=w677, f=0) -> (s? t:f=w676:i32)
                      n184 = property on="Log File" class="Path"("Value"=w669) -> ()  [unwired: 2 in, 2 out]
                      n185 = property on="Cycles" class="DigNum (strict)"("Disabled"=w676) -> ()  [unwired: 2 in, 2 out]
                      n186 = local read "Legacy Save"() -> (w673:bool)
                      n187 = case shown="True" w673 {
                        tunnel: [FALSE w708] -> w672
                        tunnel: w669 -> [_ _]
                        frame False {
                          n188 = local read "Front Panel Window:Title"() -> (w682:string)
                          n189 = property class="VI"("Front Panel Window:Title"=w682) -> ()  [unwired: 2 in, 2 out]
                        }
                        frame True {
                          (unwired) T9."new or existing file" ("select mode (2)")
                          n190 = call <vilib>:"Open Registry Key.vi"("security access mask (KEY_READ | KEY_WRITE)"=Registry_SAM."KEY_READ", "subkey"="SOFTWARE\\Microsoft\\Windows\\CurrentVersion\\Explorer\\Shell Folders\\", "root key (HKEY_LOCAL_MACHINE)"=Registry_RtKey."HKEY_LOCAL_MACHINE") -> ("error out"=w689:errorcluster, "refnum out"=w691:T10)  [unwired: 7 in]
                          n191 = call-poly <vilib>:"Read Registry Value Simple.vi"("error in (no error)"=w689, "default data"="C:\\Documents and Settings\\All Users\\Documents\\", "value"="Common Documents", "refnum"=w691) -> ("error out"=w690:errorcluster, "String/Binary data"=w697:string, "refnum out"=w692:T10)  [unwired: 2 in, 1 out]
                          n192 = call <vilib>:"Close Registry Key.vi"("error in (no error)"=w690, "refnum"=w692) -> ()  [unwired: 5 in, 1 out]
                          n193 = Concatenate Strings(w697, "\\My Gamry Data\\" ("string")) -> (w699:string)
                          n194 = String To Path(string=w699) -> (path=w687:path)
                          n195 = local read "Front Panel Window:Title"() -> (w704:string)
                          n196 = File Dialog(6:"*.txt" ("pattern"), 7:"Data File Location" ("prompt"), 9:"logfile.txt" ("default name"), 11:w687) -> (0:w684:errorcluster, 3:w685:path)  [unwired: 3 in, 2 out]
                          n197 = Unbundle(w684) -> ()  [unwired: 3 out]
                          n198 = local write "Log File"(w685) -> ()
                          n199 = call <vilib>:"Open_Create_Replace File.vi"("function (open:0)"=T6."create or replace", "file path"=w685) -> ("error out"=w709:errorcluster, "refnum"=w711:refnum<file>)  [unwired: 6 in, 2 out]
                          n200 = Path To String(path=w685) -> (string=w702:string)
                          n201 = local write "Log File Refnum"(w711) -> ()
                          n202 = Unbundle By Name(w709) -> ("status"=w706:bool)
                          n203 = Empty String/Path?(string/path=w685) -> (empty?=w707:bool)
                          n204 = Or(x=w707, y=w706) -> (x .or. y?=w708:bool)
                          n205 = Concatenate Strings(w704, " - " ("string"), w702) -> (w705:string)
                          n206 = property class="VI"("Front Panel Window:Title"=w705) -> ()  [unwired: 2 in, 2 out]
                        }
                      }
                      n207 = property class="WFChart (strict)"("History Data"=sgl[][] []) -> ()  [unwired: 2 in, 2 out]
                      n208 = property on="I vs. V" class="XYGraph (strict)"("Value"=cluster{dbl, dbl}[] [] ("I vs. V")) -> ()  [unwired: 2 in, 2 out]
                      n209 = local write "Vf History"(w670) -> ()
                      n210 = local write "Im History"(w670) -> ()
                      n211 = local write "Control Amp Overload"(w668) -> ()
                      n212 = local write "Voltage Overload"(w668) -> ()
                      n213 = local write "Current Overload"(w668) -> ()
                      n214 = case shown="True" w672 {
                        frame False {
                        }
                        frame True {
                          n215 = local write "Legacy Save"(FALSE) -> ()
                        }
                      }
                      n216 = call "Log File Error"("Enable"=w672) -> ()  [unwired: 9 in, 2 out]
                    }
                    frame "Initialize Objects" {
                      # "Register a sub VI to handle our DataAvailable and DataDone events"
                      n217 = local read "Pstat"() -> (w713:refnum<k7>)
                      n218 = invoke class="IGamryPstat" method="ModelNo"(reference=w713, error in=w712) -> (reference out=w714:refnum<k7>, error out=w715:errorcluster, "ModelNo"=w718:i32)  [unwired: 1 in]
                      n219 = Equal?(x=w718, y=4) -> (x = y?=w716:bool)
                      n220 = case shown="True" w716 {
                        tunnel: w714 -> [w734 w739]
                        tunnel: w715 -> [w733 w738]
                        tunnel: [w734 w737] -> w720
                        tunnel: [w733 w736] -> w719
                        frame False {
                        }
                        frame True {
                          n221 = invoke class="IGamryPstat" method="SetExtSrceEnable"(reference=w739, error in=w738, "ExtSrceEnable"=TRUE) -> (reference out=w737:refnum<k7>, error out=w736:errorcluster)  [unwired: 1 in, 2 out]
                        }
                      }
                      n222 = local read "CtrlMode"() -> (w725:u32)
                      n223 = invoke class="IGamryPstat" method="SetCtrlMode"(reference=w720, error in=w719, "CtrlMode"=w725) -> (reference out=w727:refnum<k7>, error out=w726:errorcluster, "SetCtrlMode"=w723:i32)  [unwired: 1 in, 1 out]
                      n224 = local write "CtrlMode"(w723) -> ()
                      n225 = local read "Dtaq"() -> (w724:refnum<k7>)
                      n226 = invoke class="IGamryDtaqIv" method="Init"(reference=w724, error in=w726, "Pstat"=w727) -> (reference out=w731:refnum<k7>, error out=w730:errorcluster)  [unwired: 1 in, 2 out]
                      n227 = control-ref of="DataDone?"() -> (w728:refnum<vi>)
                      n228 = vi-ref "DtaqDataDoneCallback - DtaqIV.vi"() -> ("vi reference"=w721:refnum<vi>)
                      n229 = node(w730, w731, w721, w728) -> (w729:refnum<k27>, w722:errorcluster)  [unwired: 1 in]
                      n230 = local write "DataDone Callback"(w729) -> ()
                      n231 = case shown="No Error" w722 {
                        tunnel: [DataAcqStates."Generate Signal" ("Data Acq States") DataAcqStates."STOP" ("Data Acq States")] -> w732
                        frame No Error {
                        }
                        frame Error {
                        }
                      }
                    }
                    frame "Generate Signal" {
                      # "Nyquist Criterion"
                      n232 = local read "Signal Frequency"() -> (w745:dbl)
                      n233 = local read "Acq. Frequency"() -> (w746:dbl)
                      n234 = local read "Signal Type"() -> (w743:u16)
                      n235 = case shown="0, 1, 3, 4" w743 {
                        tunnel: w746 -> [_ w754]
                        tunnel: w745 -> [_ w752]
                        tunnel: [TRUE w750] -> w744
                        frame Default {
                        }
                        frame 0, 1, 3, 4 {
                          n236 = Multiply(x=2.0, y=w752) -> (x*y=w753:dbl)
                          n237 = Greater?(x=w754, y=w753) -> (0:w750:bool)
                        }
                      }
                      n238 = case shown="True" w744 {
                        tunnel: w745 -> [_ w778]
                        tunnel: w746 -> [_ w762]
                        tunnel: w748 -> [w756 w770]
                        tunnel: [DataAcqStates."STOP" ("Data Acq States") w768] -> w747
                        tunnel: [w755 w759] -> w742
                        frame False {
                          n239 = call "Nyquist Criterion"("error in (no error)"=w756, "Enable"=TRUE) -> ("error out"=w755:errorcluster)  [unwired: 8 in, 1 out]
                        }
                        frame True {
                          n240 = local read "Amplitude"() -> (w779:dbl)
                          n241 = local read "Continuous"() -> (w776:bool)
                          n242 = local read "Signal Type"() -> (w775:u16)
                          n243 = local read "Cycles"() -> (w777:u32)
                          n244 = local read "Phase Offset"() -> (w781:dbl)
                          n245 = local read "Duty Cycle"() -> (w792:dbl)
                          n246 = local read "DC Offset"() -> (w780:dbl)
                          n247 = local read "Scan Rate"() -> (w782:dbl)
                          n248 = local read "Final"() -> (w783:dbl)
                          n249 = local read "Initial"() -> (w784:dbl)
                          n250 = case shown="0, 1, 4" w775 {
                            selector: w775 -> [w818 w825 w860 w870 _ _ w913 _]
                            tunnel: w776 -> [w820 w835 w862 _ _ w900 _ w931]
                            tunnel: w777 -> [w819 w834 w861 _ _ w899 _ w930]
                            tunnel: w762 -> [w809 w833 w859 w867 w887 w898 w914 w936]
                            tunnel: w778 -> [w808 _ w850 _ _ _ _ _]
                            tunnel: w779 -> [w817 _ w858 _ _ _ _ _]
                            tunnel: w780 -> [w816 _ w857 _ w882 _ _ _]
                            tunnel: w781 -> [w815 _ w856 _ _ _ _ _]
                            tunnel: w782 -> [_ w832 _ w876 _ _ w915 _]
                            tunnel: w783 -> [_ w831 _ w875 _ _ w916 _]
                            tunnel: w784 -> [_ w830 _ w874 _ _ w917 _]
                            tunnel: [w814 w828 w855 w872 w885 w895 w919 dbl[] []] -> w785
                            tunnel: [w813 w829 w854 1 ("t") -1 ("t") w896 1 ("t") w929] -> w795
                            tunnel: [w812 w827 w853 w868 w884 w897 w920 w935] -> w764
                            tunnel: [w811 w826 w852 w871 0 ("error") 0 ("error") w918 0 ("error")] -> w791
                            tunnel: w792 -> [_ _ w851 _ _ _ _ _]
                            frame 0, 1, 4 {
                              w806 = FALSE
                              # "Sine, Cosine, Sawtooth"
                              n251 = Select(t=-1, s=w820, f=w819) -> (s? t:f=w813:u32)
                              n252 = Reciprocal(x=w808) -> (1/x=w807:dbl)
                              n253 = Reciprocal(x=w809) -> (1/x=w812:dbl)
                              n254 = Multiply(x=w809, y=w807) -> (x*y=w810:dbl)
                              n255 = call <vilib>:"Signal Generator by Duration.vi"("signal type"=w818, "duration"=w807, "# of samples"=w810, "frequency"=w808, "amplitude"=w817, "dc offset"=w816, "phase in"=w815) -> ("signal"=w814:dbl[], "error"=w811:i32)  [unwired: 5 in, 2 out]
                              n256 = local write "IV_Genfilname"(w806) -> ()
                              n257 = local write "Recording IV"(w806) -> ()
                            }
                            frame 2 {
                              w822 = FALSE
                              # "Triangle"
                              n258 = Select(t=-1, s=w835, f=w834) -> (s? t:f=w829:u32)
                              n259 = Subtract(x=w831, y=w830) -> (x-y=w840:dbl)
                              n260 = Add(x=w831, y=w830) -> (x+y=w836:dbl)
                              n261 = Divide(x=w840, y=w832) -> (x/y=w845:dbl)
                              n262 = Divide(x=w840, y=2.0) -> (x/y=w839:dbl)
                              n263 = Divide(x=w836, y=2.0) -> (x/y=w838:dbl)
                              n264 = Reciprocal(x=w833) -> (1/x=w827:dbl)
                              n265 = Absolute Value(x=w845) -> (abs(x)=w844:dbl)
                              n266 = Multiply(x=w844, y=2.0) -> (x*y=w823:dbl)
                              n267 = Reciprocal(x=w823) -> (1/x=w824:dbl)
                              n268 = Multiply(x=w833, y=w823) -> (x*y=w847:dbl)
                              n269 = local write "Recording IV"(w822) -> ()
                              n270 = local write "IV_Genfilname"(w822) -> ()
                              n271 = call <vilib>:"Signal Generator by Duration.vi"("signal type"=w825, "duration"=w823, "# of samples"=w847, "frequency"=w824, "amplitude"=w839, "dc offset"=w838, "phase in"=270.0) -> ("signal"=w828:dbl[], "error"=w826:i32)  [unwired: 5 in, 2 out]
                            }
                            frame 3 {
                              w848 = FALSE
                              # "Square Wave"
                              n272 = Select(t=-1, s=w862, f=w861) -> (s? t:f=w854:u32)
                              n273 = Reciprocal(x=w850) -> (1/x=w849:dbl)
                              n274 = Reciprocal(x=w859) -> (1/x=w853:dbl)
                              n275 = Multiply(x=w859, y=w849) -> (x*y=w864:dbl)
                              n276 = call <vilib>:"Signal Generator by Duration.vi"("signal type"=w860, "duration"=w849, "# of samples"=w864, "frequency"=w850, "amplitude"=w858, "dc offset"=w857, "phase in"=w856, "square wave duty cycle (%)"=w851) -> ("signal"=w855:dbl[], "error"=w852:i32)  [unwired: 4 in, 2 out]
                              n277 = local write "Recording IV"(w848) -> ()
                              n278 = local write "IV_Genfilname"(w848) -> ()
                            }
                            frame 5, 6 {
                              w865 = TRUE
                              # "Ramp"
                              n279 = Subtract(x=w875, y=w874) -> (x-y=w878:dbl)
                              n280 = Divide(x=w878, y=w876) -> (x/y=w877:dbl)
                              n281 = Absolute Value(x=w877) -> (abs(x)=w866:dbl)
                              n282 = Reciprocal(x=w867) -> (1/x=w868:dbl)
                              n283 = Reciprocal(x=w866) -> (1/x=w869:dbl)
                              n284 = Multiply(x=w867, y=w866) -> (x*y=w880:dbl)
                              n285 = local write "IV_Genfilname"(w865) -> ()
                              n286 = local write "Recording IV"(w865) -> ()
                              n287 = call <vilib>:"Signal Generator by Duration.vi"("signal type"=w870, "duration"=w866, "# of samples"=w880, "frequency"=w869, "amplitude"=w878, "dc offset"=w874, "phase in"=0.0) -> ("signal"=w872:dbl[], "error"=w871:i32)  [unwired: 5 in, 2 out]
                            }
                            frame 7 {
                              w881 = FALSE
                              # "Single Point"
                              n288 = Reciprocal(x=w887) -> (1/x=w884:dbl)
                              n289 = Initialize Array(w882, 1 ("dimension size")) -> (w885:dbl[])
                              n290 = local write "Recording IV"(w881) -> ()
                              n291 = local write "IV_Genfilname"(w881) -> ()
                            }
                            frame 8 {
                              w889 = FALSE
                              w892 = T11 2 items=["both", "start of string", "end of string"] ("location (both)")
                              (unwired) TRUE ("convert eol (F)")
                              # "From File"
                              n292 = local read "Filename"() -> (w910:path)
                              n293 = Select(t=-1, s=w900, f=w899) -> (s? t:f=w896:u32)
                              n294 = call <vilib>:"Open_Create_Replace File.vi"("function (open:0)"=T6."open (read only)", "file path"=w910) -> ("error out"=w907:errorcluster, "file size (bytes)"=w908:i32, "new file path"=w909:path, "refnum"=w911:refnum<file>)  [unwired: 6 in]
                              n295 = local write "Filename"(w909) -> ()
                              n296 = Reciprocal(x=w898) -> (1/x=w897:dbl)
                              n297 = Read from Text File(file (use dialog)=w911, count=w908, error in=w907) -> (refnum out=w901:refnum<file>, text=w891:string, error out=w902:errorcluster)  [unwired: 1 in, 1 out]
                              n298 = local write "From File Refnum"(w901) -> ()
                              n299 = Close File(refnum=w901, error in=w902) -> ()  [unwired: 2 out]
                              n300 = local write "IV_Genfilname"(w889) -> ()
                              n301 = call <vilib>:"Trim Whitespace.vi"("string"=w891, "location (both)"=w892) -> ("trimmed string"=w890:string)
                              n302 = local write "Recording IV"(w889) -> ()
                              n303 = local write "File Data"(w890) -> ()
                              n304 = Spreadsheet String To Array(delimiter (Tab)="\n", format string="%f", spreadsheet string=w890, array type (2D Dbl)=dbl[] [] ("initialized array")) -> (array=w895:dbl[])
                            }
                            frame 9 {
                              w912 = TRUE
                              # "IV Curve"
                              n305 = Subtract(x=w916, y=w917) -> (x-y=w925:dbl)
                              n306 = Divide(x=w925, y=w915) -> (x/y=w924:dbl)
                              n307 = Absolute Value(x=w924) -> (abs(x)=w922:dbl)
                              n308 = Reciprocal(x=w914) -> (1/x=w920:dbl)
                              n309 = Reciprocal(x=w922) -> (1/x=w923:dbl)
                              n310 = Multiply(x=w914, y=w922) -> (x*y=w927:dbl)
                              n311 = local write "IV_Genfilname"(w912) -> ()
                              n312 = local write "Recording IV"(w912) -> ()
                              n313 = call <vilib>:"Signal Generator by Duration.vi"("signal type"=w913, "duration"=w922, "# of samples"=w927, "frequency"=w923, "amplitude"=w925, "dc offset"=w917, "phase in"=0.0) -> ("signal"=w919:dbl[], "error"=w918:i32)  [unwired: 5 in, 2 out]
                            }
                            frame Default {
                              w928 = FALSE
                              n314 = Reciprocal(x=w936) -> (1/x=w935:dbl)
                              n315 = Select(t=-1, s=w931, f=w930) -> (s? t:f=w929:u32)
                              n316 = local write "IV_Genfilname"(w928) -> ()
                              n317 = local write "Recording IV"(w928) -> ()
                            }
                          }
                          n318 = call <vilib>:"Error Cluster From Error Code.vi"("error in (no error)"=w770, "error code (0)"=w791) -> ("error out"=w772:errorcluster)  [unwired: 7 in]
                          n319 = property class="WFChart (strict)"("X Scale.Offset and Multiplier:Multiplier"=w764, "X Scale.Range:Minimum"=0.0, "X Scale.Range:Maximum"=10.0 ("y")) -> ()  [unwired: 2 in, 2 out]
                          n320 = local read "Log File Refnum"() -> (w794:refnum<file>)
                          n321 = local read "CtrlMode"() -> (w767:u32)
                          n322 = local read "Legacy Save"() -> (w793:bool)
                          n323 = local read "GAMRYCOMLib.IGamrySignal"() -> (w786:refnum<k7>)
                          n324 = local read "CtrlMode"() -> (w773:u32)
                          n325 = local read "Pstat"() -> (w774:refnum<k7>)
                          n326 = local read "Signal"() -> (w766:refnum<k7>)
                          n327 = case shown="True" w793 {
                            tunnel: w794 -> [_ w805]
                            tunnel: [w798 w802] -> w771
                            tunnel: w762 -> [_ w801]
                            tunnel: w772 -> [w798 w800]
                            tunnel: w767 -> [_ w799]
                            frame False {
                            }
                            frame True {
                              n328 = call "Write File Header.vi"("Curve Name"="VFPCURVE", "App Name"="VFP600", "error in"=w800, "Hz"=w801, "Control Mode"=w799, "File Refnum In"=w805) -> ("error out"=w802:errorcluster)  [unwired: 2 in, 1 out]
                            }
                          }
                          n329 = call "SigArrayInit.vi"("Signal Array"=w785, "Pstat"=w774, "Signal In"=w766, "CtrlMode"=w773, "Cycles"=w795, "Sample Rate"=w764, "error in (no error)"=w771) -> ("Pstat Out"=w789:refnum<k7>, "Signal Out"=w769:refnum<k7>, "error out"=w790:errorcluster)  [unwired: 6 in]
                          n330 = Variant To Data(error in=w790, type=w786, Variant=w769) -> (data=w787:refnum<k7>, error out=w788:errorcluster)
                          n331 = invoke class="IGamryPstat" method="SetSignal"(reference=w789, error in=w788, "Signal"=w787) -> (reference out=w761:refnum<k7>, error out=w760:errorcluster)  [unwired: 1 in, 2 out]
                          n332 = invoke class="IGamryPstat" method="InitSignal"(reference=w761, error in=w760) -> (error out=w759:errorcluster)  [unwired: 1 in, 2 out]
                          n333 = case shown="No Error" w759 {
                            tunnel: [DataAcqStates."Data Acq Setup" ("Data Acq States") DataAcqStates."STOP" ("Data Acq States")] -> w768
                            frame No Error {
                            }
                            frame Error {
                            }
                          }
                        }
                      }
                    }
                    frame "Data Acq Setup" {
                      n334 = case shown="No Error" w940 {
                        selector: w940 -> [w951 w953]
                        tunnel: [w951 w953] -> w941
                        frame No Error {
                          w952 = TRUE ("ForcePstatFunctionUpdate")
                          n335 = local write "Taking Data"(w952) -> ()
                          n336 = property on="ForcePstatFunctionUpdate" class="Bool (strict)"("Value (Signaling)"=w952) -> ()  [unwired: 2 in, 2 out]
                        }
                        frame Error {
                        }
                      }
                      n337 = local read "Auto Cell Switch"() -> (w942:bool)
                      n338 = local read "Pstat"() -> (w939:refnum<k7>)
                      n339 = case shown="True" w942 {
                        tunnel: w941 -> [w945 w950]
                        tunnel: [w945 w948] -> w938
                        tunnel: w939 -> [_ w946]
                        frame False {
                        }
                        frame True {
                          w949 = 1 items=["CellOff", "CellOn"] ("CellState")
                          n340 = local write "Cell State"(TRUE) -> ()
                          n341 = invoke class="IGamryPstat" method="SetCell"(reference=w946, error in=w950, "CellState"=w949) -> (error out=w948:errorcluster)  [unwired: 1 in, 3 out]
                        }
                      }
                      n342 = case shown="No Error" w938 {
                        tunnel: [DataAcqStates."Acquire Data" ("Data Acq States") DataAcqStates."STOP" ("Data Acq States")] -> w937
                        frame No Error {
                        }
                        frame Error {
                        }
                      }
                    }
                    frame "Acquire Data" {
                      # "Tell the Dtaq to Run"
                      n343 = local read "Dtaq"() -> (w957:refnum<k7>)
                      n344 = invoke class="IGamryDtaqIv" method="Run"(reference=w957, error in=w956, "AutoRun"=TRUE) -> (error out=w959:errorcluster)  [unwired: 1 in, 3 out]
                      n345 = while {
                        tunnel: [w1026] -> w954
                        tunnel: w959 -> [w1028]
                        stop <- w971 stop-if-true
                        # "Overload"
                        # "If we fail here, it is likely due to a device being turned off,\nas any \"Dtaq not initialized\" errors would crop up in earlier states,\nso we'll give a more helpful error."
                        # "Im"
                        # "Vf"
                        # "Take the actual data"
                        # "Poll 2x as often as axq frequency, or X ms, whichever is larger."
                        n346 = local read "Acq. Frequency"() -> (w999:dbl)
                        n347 = local read "Dtaq"() -> (w1047:refnum<k7>)
                        n348 = local read "Im History"() -> (w1023:sgl[])
                        n349 = local read "Vf History"() -> (w1024:sgl[])
                        n350 = invoke class="IGamryDtaqIv" method="Cook"(reference=w1047, error in=w1028, "NumPoints"=1024) -> (error out=w1027:errorcluster, "Data"=w1045:variant)  [unwired: 2 in, 3 out]
                        n351 = Reciprocal(x=w999) -> (1/x=w1042:dbl)
                        n352 = Multiply(x=w1042, y=1000.0) -> (x*y=w1040:dbl)
                        n353 = Divide(x=w1040, y=2.0) -> (x/y=w1038:dbl)
                        n354 = Array Size(array=w1023) -> (size(s)=w1019:i32)
                        n355 = Array Size(array=w1024) -> (size(s)=w1033:i32)
                        n356 = Subtract(x=w1019, y=16384) -> (x-y=w1021:i32)
                        n357 = Max & Min(x=w1038, y=60.0) -> (max(x,y)=w1036:dbl)  [unwired: 1 out]
                        n358 = Subtract(x=w1033, y=16384) -> (x-y=w1031:i32)
                        n359 = Array Subset(array=w1023, index=w1021) -> (w1022:sgl[])  [unwired: 1 in]
                        n360 = Array Subset(array=w1024, index=w1031) -> (w1029:sgl[])  [unwired: 1 in]
                        n361 = Variant To Data(error in=w1027, type=sgl[][] [], Variant=w1045) -> (data=w1014:sgl[][], error out=w1012:errorcluster)
                        n362 = Wait (ms)(milliseconds to wait=w1036) -> ()  [unwired: 1 out]
                        n363 = Index Array(array=w1014, index (row)=3) -> (element=w993:sgl[])  [unwired: 1 in]
                        n364 = Index Array(array=w1014, index (row)=1) -> (element=w982:sgl[])  [unwired: 1 in]
                        n365 = Index Array(array=w1014, index (row)=5) -> (element=w1013:sgl[])  [unwired: 1 in]
                        n366 = Build Array(w982, w993) -> (w994:sgl[][])
                        n367 = Build Array (concatenate)(w1022, w993) -> (w1004:sgl[])
                        n368 = Array Size(array=w1004) -> (size(s)=w1006:i32)
                        n369 = Subtract(x=w1006, y="Smoothing Parameter") -> (x-y=w1005:i32)
                        n370 = Array Subset(array=w1004, index=w1005, length="Smoothing Parameter") -> (w1003:sgl[])
                        n371 = call-poly <vilib>:"Mean.vi"("X"=w1003) -> ("mean"=w1011:dbl, "error"=w996:i32)
                        n372 = Build Array (concatenate)(w1029, w982) -> (w1007:sgl[])
                        n373 = Array Size(array=w1007) -> (size(s)=w1010:i32)
                        n374 = Subtract(x=w1010, y="Smoothing Parameter") -> (x-y=w1009:i32)
                        n375 = Array Subset(array=w1007, index=w1009, length="Smoothing Parameter") -> (w1008:sgl[])
                        n376 = call-poly <vilib>:"Mean.vi"("X"=w1008) -> ("mean"=w975:dbl)  [unwired: 1 out]
                        n377 = Divide(x=w975, y=w1011) -> (x/y=w1001:dbl)
                        n378 = local write item#33(w994) -> ()
                        n379 = local read "XY Graph Flipped?"() -> (w1017:bool)
                        n380 = Multiply(x=w996, y=1000000000) -> (x*y=w995:i32)
                        n381 = local write "Vf History"(w1007) -> ()
                        n382 = local write "Im History"(w1004) -> ()
                        n383 = Divide(x=w1001, y=1000000) -> (x/y=w990:dbl)
                        n384 = call "calculate_resistance.vi"("Bare Resistance (MOhm)"="Bare Resistance \n(MOhm)", "Live Resistance"=w990, "Solution Conductance \nS/m"="Solution Conductance", "Sealed Resistance (MOhm)"="Sealed Resistance\n(MOhm)", "Membrane Thickness (nm)"="Membrane Thickness \n(nm)", "Override"="Enable Section", "Desired Pore Size (nm)"="Desired Pore Size (nm)") -> ("Boolean"=w974:bool, "Capillary Diameter (nm)"=→"Capillary Diameter (nm)":dbl, "Target Golovochenko  (MOhm)"=→"Target Resistance (adjusted Golovochenko)  (MOhm)":dbl)  [unwired: 10 in]
                        n385 = case shown="False" w974 {
                          selector: w974 -> [w1055 w1056]
                          tunnel: [w1055 w1056] -> w973
                          frame False {
                            n386 = local write "Start/Stop Saving"(w1055) -> ()
                          }
                          frame True {
                          }
                        }
                        n387 = for {
                          tunnel: w1013 -> [w1153] mode=indexing
                          w1141 = cluster{u32, u32}[] [{7536640, 7536640}, {16744448, 16744448}]
                          w1142 = cluster{u32, u32}[] [{7536640, 7536640}, {16711680, 16711680}]
                          n388 = call "VFPOverloads.vi"("Overload IN"=w1153) -> ("Overloads"=w1147:T12)  [unwired: 9 in, 1 out]
                          n389 = Unbundle By Name(w1147) -> ("CA Overload"=w1151:bool)
                          n390 = Unbundle By Name(w1147) -> ("I Overload"=w1143:bool, "I ADC Railed"=w1146:bool)
                          n391 = Unbundle By Name(w1147) -> ("V Overload"=w1149:bool, "V ADC Railed"=w1148:bool)
                          n392 = Or(x=w1143, y=w1146) -> (x .or. y?=w1145:bool)
                          n393 = Or(x=w1149, y=w1148) -> (x .or. y?=w1150:bool)
                          n394 = local write "Control Amp Overload"(w1151) -> ()
                          n395 = Select(t=w1142, s=w1149, f=w1141) -> (s? t:f=w1152:cluster{u32, u32}[])
                          n396 = Select(t=w1142, s=w1143, f=w1141) -> (s? t:f=w1144:cluster{u32, u32}[])
                          n397 = property on="Voltage Overload" class="Bool (strict)"("Value"=w1150, "Colors [4]"=w1152) -> ()  [unwired: 2 in, 2 out]
                          n398 = property on="Current Overload" class="Bool (strict)"("Value"=w1145, "Colors [4]"=w1144) -> ()  [unwired: 2 in, 2 out]
                        }
                        n399 = local write "Current(nA)"(w995) -> ()
                        n400 = local write "Resistance (MOhm)"(w990) -> ()
                        n401 = case shown="False" w1017 {
                          tunnel: w1007 -> [w1156 w1159]
                          tunnel: w1004 -> [w1155 w1158]
                          tunnel: [w1154 w1157] -> w1018
                          frame True {
                            n402 = Build Cluster Array(w1155, w1156) -> (w1154:cluster{sgl, sgl}[])
                          }
                          frame False {
                            n403 = Build Cluster Array(w1159, w1158) -> (w1157:cluster{sgl, sgl}[])
                          }
                        }
                        n404 = local read "IV_Genfilname"() -> (w969:bool)
                        n405 = local read "DataDone?"() -> (w1048:bool)
                        n406 = local read "Start/Stop"() -> (w1050:bool)
                        n407 = local write "I vs. V"(w1018) -> ()
                        n408 = local write "Start/Stop"(w973) -> ()
                        n409 = local read "Save on Start"() -> (w964:bool)
                        n410 = Not(x=w1050) -> (.not. x?=w1049:bool)
                        n411 = call <vilib>:"Find First Error.vi"("error in (no error)"=w1012) -> ("error out"=w1025:errorcluster, "error?"=w1002:bool)  [unwired: 3 in]
                        n412 = Or(x=w1048, y=w1049) -> (x .or. y?=w1030:bool)
                        n413 = Or(x="Generate Filename", y=w969) -> (x .or. y?=w966:bool)
                        n414 = Or(x=w1002, y=w1030) -> (x .or. y?=w971:bool)
                        n415 = Or(x=w966, y=w964) -> (x .or. y?=w965:bool)
                        n416 = case shown="True" w965 {
                          tunnel: [w1112 w1116] -> w976
                          tunnel: [w1111 w1113] -> w963
                          tunnel: w964 -> [w1111 w1113]
                          frame False {
                            n417 = local read "Log File Refnum 2"() -> (w1112:refnum<file>)
                          }
                          frame True {
                            (unwired) T9."new or existing file" ("select mode (2)")
                            n418 = local write "First Run IV"(TRUE) -> ()
                            n419 = Get Date/Time In Seconds() -> (seconds since 1Jan1904=w1123:timestamp)
                            n420 = local write "IV_Genfilname"(FALSE) -> ()
                            n421 = Format Date/Time String(time format string (%c)="%d%m%y" ("pattern"), seconds (now)=w1123) -> (date/time string=w1131:string)  [unwired: 1 in]
                            n422 = Concatenate Strings("D:\\Gamry\\" ("default data"), w1131, "\\" ("pattern")) -> (w1133:string)
                            n423 = String To Path(string=w1133) -> (path=w1121:path)
                            n424 = call <vilib>:"Check if File or Folder Exists.vi"("path"=w1121) -> ("file or folder exists?"=w1120:bool)  [unwired: 8 in, 2 out]
                            "file or folder exists?" <- w1120
                            n425 = case shown="False" w1120 {
                              tunnel: w1121 -> [w1139 w1140]
                              tunnel: [w1138 w1140] -> w1122
                              frame False {
                                n426 = call "directory_structure_creator.vi"("Path to be created"=w1139) -> ("Duplicate \"Path to be created\""=w1138:path)
                              }
                              frame True {
                              }
                            }
                            n427 = Path To String(path=w1122) -> (string=w1127:string)
                            n428 = Concatenate Strings(w1127, "\\" ("pattern"), w1131, ".txt" ("pattern")) -> (w1129:string)
                            n429 = String To Path(string=w1129) -> (path=w1126:path)
                            n430 = local read "Front Panel Window:Title 2"() -> (w1135:string)
                            n431 = call <vilib>:"Create File with Incrementing Suffix.vi"("format string (\" (%d)\")"="_%d" ("pattern"), "file path"=w1126) -> ("error out"=w1118:errorcluster, "actual path"=w1117:path, "refnum out"=w1116:refnum<file>)  [unwired: 7 in]
                            "?" <- w1117
                            n432 = local write "Log File Refnum 2"(w1116) -> ()
                            n433 = local write "Log File 2"(w1117) -> ()
                            n434 = Unbundle(w1118) -> ()  [unwired: 3 out]
                            n435 = Path To String(path=w1117) -> (string=w1137:string)
                            n436 = Concatenate Strings(w1135, " - " ("string"), w1137) -> (w1134:string)
                            n437 = property class="VI"("Front Panel Window:Title"=w1134) -> ()  [unwired: 2 in, 2 out]
                          }
                        }
                        n438 = case shown="No Error" w1025 {
                          selector: w1025 -> [w1160 w1162]
                          tunnel: [w1160 w1161] -> w1026
                          frame No Error {
                          }
                          frame Error {
                            n439 = Bundle By Name(cluster=w1162, "source"="Data Acq\n\nPlease confirm that your device has \nnot been disabled or disconnected.") -> (w1161:errorcluster)
                          }
                        }
                        n440 = local read "Log File Refnum"() -> (w1034:refnum<file>)
                        n441 = local read "Legacy Save"() -> (w1035:bool)
                        n442 = case shown="True" w1035 {
                          tunnel: w1034 -> [_ w1169]
                          tunnel: w994 -> [_ w1165]
                          frame False {
                          }
                          frame True {
                            n443 = Transpose 2D Array(2D array=w1165) -> (transposed array=w1166:sgl[][])
                            n444 = Array To Spreadsheet String(array=w1166, 3:"%5g" ("format string")) -> (spreadsheet string=w1168:string)  [unwired: 1 in]
                            n445 = Write to Binary File(file (use dialog)=w1169, data=w1168, 5:FALSE ("prepend array or string size? (T)")) -> ()  [unwired: 3 in, 3 out]
                          }
                        }
                        n446 = property on="Recording IV" class="Bool (strict)"() -> ("Value"=w972:bool)  [unwired: 2 in, 2 out]
                        n447 = case shown="True" w972 {
                          tunnel: w982 -> [w1075 w1083]
                          tunnel: w993 -> [w1076 w1080]
                          tunnel: [w1075 w1079] -> w992
                          tunnel: [w1076 w1078] -> w991
                          frame False {
                          }
                          frame True {
                            n448 = local read "First Run IV"() -> (w1077:bool)
                            n449 = feedback #1() -> (w1081:sgl[])  [unwired: 1 in]
                            n450 = Build Array (concatenate)(w1081, w1080) -> (w1078:sgl[])
                            n451 = feedback-in #1(w1078) -> ()
                            n452 = feedback #2() -> (w1082:sgl[])  [unwired: 1 in]
                            n453 = Build Array (concatenate)(w1082, w1083) -> (w1079:sgl[])
                            n454 = feedback-in #2(w1079) -> ()
                            n455 = case shown="True" w1077 {
                              frame False {
                              }
                              frame True {
                                n456 = call <vilib>:"High Resolution Relative Seconds.vi"() -> ("relative seconds"=→"IV_start":dbl)
                                n457 = local write "Start/Stop Saving"(TRUE) -> ()
                                n458 = local write "First Run IV"(FALSE) -> ()
                              }
                            }
                          }
                        }
                        n459 = local read "Start/Stop Saving"() -> (w980:bool)
                        n460 = case shown="True" w980 {
                          tunnel: w994 -> [_ w1107]
                          tunnel: w976 -> [_ w1105]
                          frame False {
                          }
                          frame True {
                            n461 = Transpose 2D Array(2D array=w1107) -> (transposed array=w1108:sgl[][])
                            n462 = Array To Spreadsheet String(array=w1108, 3:"%5g" ("format string")) -> (spreadsheet string=w1110:string)  [unwired: 1 in]
                            n463 = Write to Binary File(file (use dialog)=w1105, data=w1110, 5:FALSE ("prepend array or string size? (T)")) -> ()  [unwired: 3 in, 3 out]
                            n464 = local write "Saving"(TRUE) -> ()
                          }
                        }
                        n465 = case shown="True" w972 {
                          tunnel: w992 -> [w1087 w1089]
                          tunnel: w991 -> [w1088 w1090]
                          tunnel: [w1087 w1090] -> w968
                          tunnel: [w1088 w1089] -> w967
                          frame False {
                          }
                          frame True {
                            n466 = local read "Initial"() -> (w1101:dbl)
                            n467 = local read "Final"() -> (w1100:dbl)
                            n468 = Absolute Value(x=w1100) -> (abs(x)=w1098:dbl)
                            n469 = Absolute Value(x=w1101) -> (abs(x)=w1097:dbl)
                            n470 = Add(x=w1098, y=w1097) -> (x+y=w1096:dbl)
                            n471 = local read "Scan Rate"() -> (w1092:dbl)
                            n472 = Absolute Value(x=w1096) -> (abs(x)=w1093:dbl)
                            n473 = local read "IV_start"() -> (w1099:dbl)
                            n474 = Divide(x=w1093, y=w1092) -> (x/y=w1091:dbl)
                            n475 = Add(x=w1099, y=w1091) -> (x+y=w1102:dbl)
                            "Done Time" <- w1102
                            n476 = call <vilib>:"High Resolution Relative Seconds.vi"() -> ("relative seconds"=w1103:dbl)
                            "Current Time" <- w1103
                            n477 = Greater Or Equal?(x=w1103, y=w1102) -> (x >= y?=w1095:bool)
                            n478 = Not(x=w1095) -> (.not. x?=w1094:bool)
                            n479 = local write "Start/Stop Saving"(w1094) -> ()
                          }
                        }
                        n480 = local read "Saving"() -> (w979:bool)
                        n481 = Not(x=w980) -> (.not. x?=w978:bool)
                        n482 = case shown="True" w963 {
                          frame False {
                          }
                          frame True {
                            n483 = local write "Start/Stop Saving"(TRUE) -> ()
                            n484 = local write "Save on Start"(FALSE) -> ()
                          }
                        }
                        n485 = And(x=w979, y=w978) -> (x .and. y?=w977:bool)
                        n486 = case shown="True" w977 {
                          tunnel: w976 -> [_ w1074]
                          tunnel: w968 -> [_ w1067]
                          tunnel: w967 -> [_ w1061]
                          frame False {
                          }
                          frame True {
                            n487 = Close File(refnum=w1074) -> ()  [unwired: 1 in, 2 out]
                            n488 = local write "Saving"(FALSE) -> ()
                            n489 = call <vilib>:"Linear Fit.vi"("Y"=w1067, "X"=w1061) -> ("Best Linear Fit"=w1057:dbl[], "slope"=w1072:dbl)  [unwired: 9 in, 3 out]
                            n490 = Multiply(x=w1072, y=100000000) -> (x*y=→"Rough Resistance (MOhm)":dbl)
                            n491 = Multiply(x=1000000000, y=w1067) -> (x*y=w1065:sgl[])
                            n492 = Multiply(x=1000000000, y=w1057) -> (x*y=w1058:dbl[])
                            n493 = call "Convert to Dynamic Data"("Array"=w1065) -> ("Dynamic Data Type"=w1064:dynamicdata)  [unwired: 3 in]
                            n494 = Bundle("type"=w1061, w1058) -> (→"Line of Best Fit":cluster{"type":sgl[], dbl[]})  [unwired: 1 in]
                            n495 = call "Convert to Dynamic Data2"("Array"=w1061) -> ("Dynamic Data Type"=w1068:dynamicdata)  [unwired: 3 in]
                            n496 = call "Build XY Graph"("Y Input"=w1064, "X Input"=w1068) -> ("XY Graph"=→"IV Data":cluster{"X":dbl[], "Y":dbl[]}[])  [unwired: 8 in, 1 out]
                            n497 = property on="IV Data" class="XYGraph (strict)"("Plot.Plot Color"=u32 0) -> ()  [unwired: 2 in, 2 out]
                            n498 = property on="IV Data" class="XYGraph (strict)"("Plot.Line Width"=2) -> ()  [unwired: 2 in, 2 out]
                          }
                        }
                        n499 = case shown="True" "Clear Graphs" {
                          frame False {
                          }
                          frame True {
                            n500 = property on="IV Data" class="XYGraph (strict)"("Value"=cluster{"X":dbl[], "Y":dbl[]}[] [] ("IV Data")) -> ()  [unwired: 2 in, 2 out]
                            n501 = property on="Line of Best Fit" class="XYGraph (strict)"("Value"=cluster{"type":sgl[], "Best Linear Fit":dbl[]} {"type"=[], "Best Linear Fit"=[]} ("Line of Best Fit")) -> ()  [unwired: 2 in, 2 out]
                          }
                        }
                      }
                      n502 = case shown="No Error" w954 {
                        tunnel: [DataAcqStates."Cleanup" ("Data Acq States") DataAcqStates."STOP" ("Data Acq States")] -> w955
                        frame No Error {
                        }
                        frame Error {
                        }
                      }
                    }
                    frame "Cleanup" {
                      n503 = local read "Auto Cell Switch"() -> (w1179:bool)
                      n504 = local read "Device Gone"() -> (w1177:bool)
                      n505 = local read "Pstat"() -> (w1175:refnum<k7>)
                      n506 = Not(x=w1177) -> (.not. x?=w1180:bool)
                      n507 = And(x=w1179, y=w1180) -> (x .and. y?=w1181:bool)
                      n508 = case shown="True" w1181 {
                        tunnel: [w1195 w1200] -> w1182
                        tunnel: w1176 -> [w1195 w1198]
                        tunnel: w1175 -> [_ w1197]
                        frame False {
                        }
                        frame True {
                          w1196 = 0 items=["CellOff", "CellOn"] ("CellState")
                          n509 = local write "Cell State"(FALSE) -> ()
                          n510 = invoke class="IGamryPstat" method="SetCell"(reference=w1197, error in=w1198, "CellState"=w1196) -> (error out=w1200:errorcluster)  [unwired: 1 in, 3 out]
                        }
                      }
                      n511 = local read "Dtaq"() -> (w1178:refnum<k7>)
                      n512 = invoke class="IGamryDtaqIv" method="Stop"(reference=w1178, error in=w1182) -> (reference out=w1172:refnum<k7>, error out=w1171:errorcluster)  [unwired: 1 in, 1 out]
                      n513 = while {
                        shift-right: [w1184] -> _
                        shift-left: w1172 -> [w1189]
                        shift-right: [w1185] -> w1170
                        shift-left: w1171 -> [w1188]
                        stop <- w1186 stop-if-true
                        n514 = invoke class="IGamryDtaqIv" method="Cook"(reference=w1189, error in=w1188, "NumPoints"=1024) -> (reference out=w1184:refnum<k7>, error out=w1185:errorcluster, "NumPoints"=w1187:i32)  [unwired: 2 in, 2 out]
                        n515 = Equal To 0?(x=w1187) -> (x = 0?=w1186:bool)
                      }
                      n516 = case shown="No Error" w1170 {
                        selector: w1170 -> [w1191 w1192]
                        tunnel: [w1191 w1192] -> w1173
                        frame No Error {
                          n517 = local write "Taking Data"(FALSE) -> ()
                        }
                        frame Error {
                        }
                      }
                      n518 = case shown="No Error" w1173 {
                        tunnel: [DataAcqStates."STOP" ("Data Acq States") DataAcqStates."STOP" ("Data Acq States")] -> w1174
                        frame No Error {
                        }
                        frame Error {
                        }
                      }
                    }
                    frame "STOP" {
                      w1207 = u8 0 ("Disabled")
                      w1202 = FALSE
                      w1210 = FALSE ("Begin")
                      # "Enable menu items"
                      # "Reset Buttons"
                      n519 = property class="App"() -> ("Application:Kind"=w1208:T13)  [unwired: 2 in, 2 out]
                      n520 = local read "Legacy Save"() -> (w1217:bool)
                      n521 = case shown="\"Run Time System\", Default" w1208 {
                        tunnel: [w1220 w1221] -> w1209
                        frame "Development System" {
                          w1220 = T14 1 items=["no dialog", "OK message", "continue or stop message", "OK message + warnings", "continue/stop + warnings"] ("type of dialog (OK msg:1)")
                        }
                        frame "Run Time System", Default {
                          w1221 = T14 1 items=["no dialog", "OK message", "continue or stop message", "OK message + warnings", "continue/stop + warnings"] ("type of dialog (OK msg:1)")
                        }
                      }
                      n522 = local read "[user-defined descriptions]"() -> (w1211:string[])
                      n523 = local write "Start/Stop"(w1210) -> ()
                      n524 = local write "DataDone?"(w1210) -> ()
                      n525 = local write "Device Gone"(w1210) -> ()
                      n526 = local read "[user-defined codes]"() -> (w1203:u32[])
                      n527 = case shown="True" w1217 {
                        tunnel: [w1226 w1228] -> w1214
                        tunnel: w1213 -> [w1226 w1227]
                        frame False {
                        }
                        frame True {
                          n528 = local read "Log File Refnum"() -> (w1229:refnum<file>)
                          n529 = Close File(refnum=w1229, error in=w1227) -> (error out=w1228:errorcluster)  [unwired: 1 out]
                        }
                      }
                      n530 = local read "DataDone Callback"() -> (w1215:refnum<k27>)
                      n531 = local write "Control Amp Overload"(w1202) -> ()
                      n532 = local write "Voltage Overload"(w1202) -> ()
                      n533 = local write "Current Overload"(w1202) -> ()
                      n534 = Not A Number/Path/Refnum?(number/path/refnum=w1215) -> (NaN/Path/Refnum?=w1216:bool)
                      n535 = case shown="False" w1216 {
                        tunnel: w1215 -> [w1224 _]
                        tunnel: w1214 -> [w1223 w1225]
                        tunnel: [w1222 w1225] -> w1205
                        frame False {
                          n536 = Unregister For Events(event registration refnum=w1224, error in=w1223) -> (error out=w1222:errorcluster)
                        }
                        frame True {
                        }
                      }
                      n537 = property on="Device" class="Ring (strict)"("Disabled"=w1207) -> ()  [unwired: 2 in, 2 out]
                      n538 = property on="CtrlMode" class="Ring (strict)"("Disabled"=w1207) -> ()  [unwired: 2 in, 2 out]
                      n539 = property on="Acq. Frequency" class="DigNum (strict)"("Disabled"=w1207) -> ()  [unwired: 2 in, 2 out]
                      n540 = call <vilib>:"General Error Handler.vi"("[user-defined codes]"=w1203, "[user-defined descriptions]"=w1211, "type of dialog (OK msg:1)"=w1209, "error in (no error)"=w1205) -> ("error out"=w1204:errorcluster)  [unwired: 7 in, 4 out]
                      n541 = property on="Vch Range" class="Ring (strict)"("Disabled"=w1207) -> ()  [unwired: 2 in, 2 out]
                      n542 = property on="Ich Range" class="Ring (strict)"("Disabled"=w1207) -> ()  [unwired: 2 in, 2 out]
                      n543 = property on="Legacy Save" class="Bool (strict)"("Disabled"=w1207) -> ()  [unwired: 2 in, 2 out]
                      n544 = local write "Start/Stop Saving"(FALSE ("Start/Stop Saving")) -> ()
                      n545 = local read "CtrlMode"() -> (w1206:u32)
                      n546 = case shown="1, Default" w1206 {
                        frame 1, Default {
                          w1218 = u8 0 ("Disabled")
                          n547 = property on="I/E Range" class="Ring (strict)"("Disabled"=w1218) -> ()  [unwired: 2 in, 2 out]
                          n548 = property on="I/E Autorange" class="Bool (strict)"("Disabled"=w1218) -> ()  [unwired: 2 in, 2 out]
                        }
                        frame 0 {
                          w1219 = u8 2 ("Disabled")
                          n549 = property on="I/E Range" class="Ring (strict)"("Disabled"=w1219) -> ()  [unwired: 2 in, 2 out]
                          n550 = property on="I/E Autorange" class="Bool (strict)"("Disabled"=w1219) -> ()  [unwired: 2 in, 2 out]
                        }
                      }
                    }
                  }
                  n551 = Equal?(x=w665, y=DataAcqStates."STOP" ("Data Acq States")) -> (x = y?=w666:bool)
                  n552 = Wait (ms)(milliseconds to wait=u32 150) -> ()  [unwired: 1 out]
                }
              }
            }
          }
          event Timeout {
            n553 = event-data() -> ()  [unwired: 1 in, 3 out]
          }
        }
        n554 = local read "Close"() -> (w656:bool)
        n555 = Not(x=w656) -> (.not. x?=w655:bool)
      }
      n556 = while {
        stop <- w164 continue-if-true
        n557 = local read "milliseconds to wait"() -> (w163:u32)
        n558 = event shown="[3] \"CtrlMode\", \"I/E Range\", \"Vch Range\", \"Ich Range\", \"Vch Filter\", \"Ich Filter\", \"I/E Autorange\", \"Vch Autorange\", \"Ich Autorange\", \"Vch Offset\", \"Ich Offset\", \"VchOffsetEnable\", \"IchOffsetEnable\", \"ForcePstatFunctionUpdate\", \"I/E Stability\", \"CA Speed\": Value Change" {
          selector: _ -> [_ _ _ _ _ _ _ _]
          dyn-events: _ -> [_ _ _ _ _ _ _ _]
          timeout: w163 -> [_ _ _ _ _ _ _ _]
          event Timeout {
            w167 = u32 2 items=["Galvanostat", "Potentiostat", "ZRA"] ("CtrlMode")
            n559 = event-data() -> ()  [unwired: 1 in, 2 out]
            n560 = local read "Taking Data"() -> (w176:bool)
            n561 = case shown="True" w176 {
              frame False {
              }
              frame True {
                n562 = local read "Pstat"() -> (w177:refnum<k7>)
                n563 = local read "Vch Autorange"() -> (w179:bool)
                n564 = local read "Ich Autorange"() -> (w180:bool)
                n565 = local read "I/E Autorange"() -> (w178:bool)
                n566 = case shown="False" w180 {
                  tunnel: w177 -> [_ w201]
                  frame False {
                    n567 = property on="Ich Range" class="Ring (strict)"("Disabled"=0) -> ()  [unwired: 2 in, 2 out]
                  }
                  frame True {
                    n568 = invoke class="IGamryPstat" method="IchRange"(reference=w201) -> ("IchRange"=w200:i32)  [unwired: 2 in, 2 out]
                    n569 = property on="Ich Range" class="Ring (strict)"("Value"=w200, "Disabled"=1) -> ()  [unwired: 2 in, 2 out]
                  }
                }
                n570 = case shown="False" w179 {
                  tunnel: w177 -> [_ w197]
                  frame False {
                    n571 = property on="Vch Range" class="Ring (strict)"("Disabled"=0) -> ()  [unwired: 2 in, 2 out]
                  }
                  frame True {
                    n572 = invoke class="IGamryPstat" method="VchRange"(reference=w197) -> ("VchRange"=w196:i32)  [unwired: 2 in, 2 out]
                    n573 = property on="Vch Range" class="Ring (strict)"("Value"=w196, "Disabled"=1) -> ()  [unwired: 2 in, 2 out]
                  }
                }
                n574 = case shown="True" w178 {
                  tunnel: w177 -> [_ w193]
                  frame False {
                    n575 = local read "CtrlMode"() -> (w181:u32)
                    n576 = case shown="1, Default" w181 {
                      frame 1, Default {
                        w182 = u8 0 ("Disabled")
                        n577 = property on="I/E Range" class="Ring (strict)"("Disabled"=w182) -> ()  [unwired: 2 in, 2 out]
                        n578 = property on="I/E Autorange" class="Bool (strict)"("Disabled"=w182) -> ()  [unwired: 2 in, 2 out]
                      }
                      frame 0 {
                        w183 = u8 2 ("Disabled")
                        n579 = property on="I/E Range" class="Ring (strict)"("Disabled"=w183) -> ()  [unwired: 2 in, 2 out]
                        n580 = property on="I/E Autorange" class="Bool (strict)"("Disabled"=w183) -> ()  [unwired: 2 in, 2 out]
                      }
                    }
                  }
                  frame True {
                    w188 = u32 0 items=["Galvanostat", "Potentiostat", "ZRA"] ("CtrlMode")
                    n581 = local read "CtrlMode"() -> (w189:u32)
                    n582 = local read "First I/E Range"() -> (w190:i32)
                    n583 = invoke class="IGamryPstat" method="IERange"(reference=w193) -> ("IERange"=w191:i32)  [unwired: 2 in, 2 out]
                    n584 = Equal?(x=w189, y=w188) -> (x = y?=w187:bool)
                    n585 = Select(t=2, s=w187, f=1) -> (s? t:f=w184:i32)
                    n586 = Subtract(x=w191, y=w190) -> (x-y=w192:i32)
                    n587 = property on="I/E Range" class="Ring (strict)"("Value"=w192, "Disabled"=w184) -> ()  [unwired: 2 in, 2 out]
                  }
                }
              }
            }
            n588 = local read "CtrlMode"() -> (w166:u32)
            n589 = local read "Family"() -> (w168:string)
            n590 = Equal?(x=w166, y=w167) -> (x = y?=w170:bool)
            n591 = Equal?(x=w168, y="PC5") -> (x = y?=w171:bool)
            n592 = And(x=w170, y=w171) -> (x .and. y?=w172:bool)
            n593 = Select(t=i32[] [0], s=w172, f=i32[] []) -> (s? t:f=w174:i32[])
            n594 = property on="CA Speed" class="Ring (strict)"("Disabled Items []"=w174) -> ()  [unwired: 2 in, 2 out]
          }
          event "Select Graph": Value Change {
            n595 = event-data() -> ("NewVal"=w202:u16)  [unwired: 1 in]
            n596 = case shown="1" w202 {
              frame 0, Default {
                n597 = property class="WFChart (strict)"("Visible"=TRUE) -> ()  [unwired: 2 in, 2 out]
                n598 = property on="I vs. V" class="XYGraph (strict)"("Visible"=FALSE) -> ()  [unwired: 2 in, 2 out]
              }
              frame 1 {
                n599 = local write "XY Graph Flipped?"(FALSE ("XY Graph Flipped?")) -> ()
                n600 = property class="WFChart (strict)"("Visible"=FALSE) -> ()  [unwired: 2 in, 2 out]
                n601 = local read "Taking Data"() -> (w205:bool)
                n602 = case shown="False" w205 {
                  frame False {
                    n603 = local read "Im History"() -> (w214:sgl[])
                    n604 = local read "Vf History"() -> (w215:sgl[])
                    n605 = Build Cluster Array(w215, w214) -> (w213:cluster{sgl, sgl}[])
                    n606 = local write "I vs. V"(w213) -> ()
                  }
                  frame True {
                  }
                }
                n607 = property on="I vs. V" class="XYGraph (strict)"("Visible"=TRUE, "X Scale.Name Label.Text"="Voltage (V)", "Y Scale.Name Label.Text"="Current (A)", "Transpose Array"=FALSE, "Plot.Plot Name"="I vs. V") -> ()  [unwired: 2 in, 2 out]
              }
              frame 2 {
                n608 = local write "XY Graph Flipped?"(TRUE ("XY Graph Flipped?")) -> ()
                n609 = property class="WFChart (strict)"("Visible"=FALSE) -> ()  [unwired: 2 in, 2 out]
                n610 = local read "Taking Data"() -> (w216:bool)
                n611 = case shown="False" w216 {
                  frame False {
                    n612 = local read "Im History"() -> (w225:sgl[])
                    n613 = local read "Vf History"() -> (w226:sgl[])
                    n614 = Build Cluster Array(w225, w226) -> (w224:cluster{sgl, sgl}[])
                    n615 = local write "I vs. V"(w224) -> ()
                  }
                  frame True {
                  }
                }
                n616 = property on="I vs. V" class="XYGraph (strict)"("Visible"=TRUE, "X Scale.Name Label.Text"="Current (A)", "Y Scale.Name Label.Text"="Voltage (V)", "Transpose Array"=FALSE, "Plot.Plot Name"="V vs. I") -> ()  [unwired: 2 in, 2 out]
              }
            }
          }
          event "Cell State": Value Change {
            n617 = event-data() -> ("NewVal"=w228:bool)  [unwired: 1 in, 5 out]
            n618 = local read "Device Open"() -> (w227:bool)
            n619 = case shown="True" w227 {
              tunnel: w228 -> [_ w231]
              frame False {
              }
              frame True {
                # "Monitor Cell Switch"
                n620 = local read "Pstat"() -> (w233:refnum<k7>)
                n621 = Boolean To (0,1)(Boolean=w231) -> (0, 1=w232:i16)
                n622 = invoke class="IGamryPstat" method="SetCell"(reference=w233, "CellState"=w232) -> ("SetCell"=w229:i32)  [unwired: 2 in, 3 out]
                n623 = Not Equal To 0?(x=w229) -> (x != 0?=→"SetCell":bool)
                "Cell Val Change NewVal" <- w231
              }
            }
          }
          event "CtrlMode", "I/E Range", "Vch Range", "Ich Range", "Vch Filter", "Ich Filter", "I/E Autorange", "Vch Autorange", "Ich Autorange", "Vch Offset", "Ich Offset", "VchOffsetEnable", "IchOffsetEnable", "ForcePstatFunctionUpdate", "I/E Stability", "CA Speed": Value Change {
            # "Adjust unit labels\naccording to\nControl Mode"
            n624 = local read "CtrlMode"() -> (w238:u32)
            n625 = event-data() -> ("CtlRef"=w235:refnum<vi>)  [unwired: 1 in]
            n626 = control-ref of="CtrlMode"() -> (w237:refnum<vi>)
            n627 = local read "Device Open"() -> (w243:bool)
            n628 = local read "Pstat"() -> (w242:refnum<k7>)
            n629 = To More Generic Class(target class=w235, reference=w237) -> (generic class reference=w236:refnum<vi>)
            n630 = Equal?(x=w235, y=w236) -> (x = y?=w239:bool)
            n631 = case shown="True" w239 {
              tunnel: w238 -> [_ w247]
              tunnel: [errorcluster {"status"=FALSE, "code"=0, "source"=""} ("error out") w246] -> w234
              frame False {
              }
              frame True {
                n632 = case shown="1, Default" w247 {
                  selector: w247 -> [_ w262]
                  tunnel: [w248 w267] -> w246
                  frame 0 {
                    w249 = u8 2 ("Disabled")
                    w251 = u16 0 items=["Fast", "Medium Fast", "Normal", "Slow"] ("I/E Stability")
                    w253 = "A" ("Caption.Text")
                    n633 = property on="Amplitude" class="DigNum (strict)"("Caption.Text"=w253) -> ()  [unwired: 2 in, 2 out]
                    n634 = property on="Scan Rate" class="DigNum (strict)"("Caption.Text"="A/s") -> ()  [unwired: 2 in, 2 out]
                    n635 = property on="DC Offset" class="DigNum (strict)"("Caption.Text"=w253) -> ()  [unwired: 2 in, 2 out]
                    n636 = property on="Final" class="DigNum (strict)"("Caption.Text"=w253) -> ()  [unwired: 2 in, 2 out]
                    n637 = property on="Initial" class="DigNum (strict)"("Caption.Text"=w253) -> ()  [unwired: 2 in, 2 out]
                    n638 = property on="I/E Stability" class="Ring (strict)"("Disabled"=u8 2, "Value"=w251) -> ()  [unwired: 2 in, 2 out]
                    n639 = property on="I/E Range" class="Ring (strict)"("Disabled"=w249) -> ()  [unwired: 2 in, 2 out]
                    n640 = property on="I/E Autorange" class="Bool (strict)"("Disabled"=w249, "Value"=TRUE) -> (error out=w248:errorcluster)  [unwired: 2 in, 1 out]
                  }
                  frame 1, Default {
                    w264 = u32 2 items=["Galvanostat", "Potentiostat", "ZRA"] ("CtrlMode")
                    w268 = u8 0 ("Disabled")
                    w270 = "V" ("Caption.Text")
                    n641 = local read "CA Speed"() -> (w256:u16)
                    n642 = local read "Family"() -> (w265:string)
                    n643 = Equal?(x=w262, y=w264) -> (x = y?=w263:bool)
                    n644 = Equal?(x=w265, y="PC5") -> (x = y?=w261:bool)
                    n645 = Equal?(x=w256, y=u16 0) -> (x = y?=w259:bool)
                    n646 = Compound Arithmetic op=AND(w263, w261, w259) -> (w258:bool)
                    n647 = Select(t=u16 1, s=w258, f=w256) -> (s? t:f=w257:u16)
                    n648 = local write "CA Speed"(w257) -> ()
                    n649 = property on="Amplitude" class="DigNum (strict)"("Caption.Text"=w270) -> ()  [unwired: 2 in, 2 out]
                    n650 = property on="Scan Rate" class="DigNum (strict)"("Caption.Text"="V/s") -> ()  [unwired: 2 in, 2 out]
                    n651 = property on="DC Offset" class="DigNum (strict)"("Caption.Text"=w270) -> ()  [unwired: 2 in, 2 out]
                    n652 = property on="Final" class="DigNum (strict)"("Caption.Text"=w270) -> ()  [unwired: 2 in, 2 out]
                    n653 = property on="Initial" class="DigNum (strict)"("Caption.Text"=w270) -> ()  [unwired: 2 in, 2 out]
                    n654 = property on="I/E Stability" class="Ring (strict)"("Disabled"=u8 0) -> ()  [unwired: 2 in, 2 out]
                    n655 = property on="I/E Range" class="Ring (strict)"("Disabled"=w268) -> ()  [unwired: 2 in, 2 out]
                    n656 = property on="I/E Autorange" class="Bool (strict)"("Disabled"=w268) -> (error out=w267:errorcluster)  [unwired: 2 in, 1 out]
                  }
                }
              }
            }
            n657 = case shown="True" w243 {
              tunnel: w242 -> [_ w278]
              tunnel: [errorcluster {"status"=FALSE, "code"=0, "source"=""} ("error out") w285] -> w240
              tunnel: w234 -> [_ w274]
              frame False {
              }
              frame True {
                w317 = 0 items=["StabilityFast", "StabilityMedFast", "StabilityNorm", "StabilitySlow"] ("Stability")
                w320 = 0 items=["GstatMode", "PstatMode", "ZRAMode", "FRAMode"] ("SetCtrlMode")
                n658 = local read "CtrlMode"() -> (w338:u32)
                n659 = local read "Ich Autorange"() -> (w327:bool)
                n660 = local read "IchOffsetEnable"() -> (w309:bool)
                n661 = local read "Ich Filter"() -> (w305:u16)
                n662 = local read "Ich Range"() -> (w336:u16)
                n663 = invoke class="IGamryPstat" method="SetCtrlMode"(reference=w278, error in=w274, "CtrlMode"=w338) -> (reference out=w314:refnum<k7>, error out=w315:errorcluster, "SetCtrlMode"=w319:i32)  [unwired: 1 in, 1 out]
                n664 = invoke class="IGamryPstat" method="SetIchFilter"(reference=w278, "Filter"=w305) -> (reference out=w302:refnum<k7>, error out=w301:errorcluster, "SetIchFilter"=w306:i32)  [unwired: 2 in, 1 out]
                n665 = invoke class="IGamryPstat" method="SetIchRange"(reference=w278, "Range"=w336) -> (reference out=w297:refnum<k7>, error out=w298:errorcluster, "SetIchRange"=w337:i32)  [unwired: 2 in, 1 out]
                n666 = invoke class="IGamryPstat" method="SetIchRangeMode"(reference=w278, "RangeMode"=w327) -> (reference out=w293:refnum<k7>, error out=w294:errorcluster, "SetIchRangeMode"=w328:bool)  [unwired: 2 in, 1 out]
                n667 = local write "CtrlMode"(w319) -> ()
                n668 = invoke class="IGamryPstat" method="SetIchOffsetEnable"(reference=w278, "OffsetEnable"=w309) -> (reference out=w299:refnum<k7>, error out=w300:errorcluster, "SetIchOffsetEnable"=w310:bool)  [unwired: 2 in, 1 out]
                n669 = local write "Ich Autorange"(w328) -> ()
                n670 = local write "IchOffsetEnable"(w310) -> ()
                n671 = local write "Ich Range"(w337) -> ()
                n672 = local write "Ich Filter"(w306) -> ()
                n673 = local read "I/E Stability"() -> (w318:u16)
                n674 = local read "Vch Range"() -> (w334:u16)
                n675 = local read "Vch Autorange"() -> (w325:bool)
                n676 = local read "Vch Filter"() -> (w304:u16)
                n677 = local read "VchOffsetEnable"() -> (w307:bool)
                n678 = Equal?(x=w319, y=w320) -> (x = y?=w321:bool)
                n679 = invoke class="IGamryPstat" method="SetVchFilter"(reference=w302, error in=w301, "Filter"=w304) -> (error out=w288:errorcluster, "SetVchFilter"=w303:i32)  [unwired: 1 in, 2 out]
                n680 = invoke class="IGamryPstat" method="SetVchRange"(reference=w297, error in=w298, "Range"=w334) -> (reference out=w295:refnum<k7>, error out=w296:errorcluster, "SetVchRange"=w335:i32)  [unwired: 1 in, 1 out]
                n681 = invoke class="IGamryPstat" method="SetVchRangeMode"(reference=w293, error in=w294, "RangeMode"=w325) -> (reference out=w291:refnum<k7>, error out=w292:errorcluster, "SetVchRangeMode"=w326:bool)  [unwired: 1 in, 1 out]
                n682 = Select(t=w317, s=w321, f=w318) -> (s? t:f=w316:i32)
                n683 = local write "Vch Range"(w335) -> ()
                n684 = local write "Vch Autorange"(w326) -> ()
                n685 = local write "Vch Filter"(w303) -> ()
                n686 = invoke class="IGamryPstat" method="SetVchOffsetEnable"(reference=w299, error in=w300, "OffsetEnable"=w307) -> (reference out=w277:refnum<k7>, error out=w276:errorcluster, "SetVchOffsetEnable"=w308:bool)  [unwired: 1 in, 1 out]
                n687 = invoke class="IGamryPstat" method="SetIEStability"(reference=w314, error in=w315, "Stability"=w316) -> (reference out=w311:refnum<k7>, error out=w312:errorcluster, "SetIEStability"=w322:i32)  [unwired: 1 in, 1 out]
                n688 = local write "VchOffsetEnable"(w308) -> ()
                n689 = local write "I/E Stability"(w322) -> ()
                n690 = local read "I/E Range"() -> (w329:u16)
                n691 = local read "First I/E Range"() -> (w330:i32)
                n692 = local read "I/E Autorange"() -> (w323:bool)
                n693 = local read "Ich Offset"() -> (w283:sgl)
                n694 = local read "CA Speed"() -> (w273:u16)
                n695 = Add(x=w329, y=w330) -> (x+y=w332:i32)
                n696 = invoke class="IGamryPstat" method="SetIERangeMode"(reference=w291, error in=w292, "RangeMode"=w323) -> (error out=w286:errorcluster, "SetIERangeMode"=w324:bool)  [unwired: 1 in, 2 out]
                n697 = local write "I/E Autorange"(w324) -> ()
                n698 = invoke class="IGamryPstat" method="SetIERange"(reference=w295, error in=w296, "Range"=w332) -> (error out=w287:errorcluster, "SetIERange"=w333:i32)  [unwired: 1 in, 2 out]
                n699 = invoke class="IGamryPstat" method="SetIchOffset"(reference=w277, error in=w276, "Offset"=w283) -> (reference out=w280:refnum<k7>, error out=w279:errorcluster, "SetIchOffset"=w284:sgl)  [unwired: 1 in, 1 out]
                n700 = invoke class="IGamryPstat" method="SetCASpeed"(reference=w311, error in=w312, "CASpeed"=w273) -> (error out=w289:errorcluster, "SetCASpeed"=w313:i32)  [unwired: 1 in, 2 out]
                n701 = local write "Ich Offset"(w284) -> ()
                n702 = local write "CA Speed"(w313) -> ()
                n703 = Subtract(x=w333, y=w330) -> (x-y=w331:i32)
                n704 = local read "Vch Offset"() -> (w282:sgl)
                n705 = local write "I/E Range"(w331) -> ()
                n706 = invoke class="IGamryPstat" method="SetVchOffset"(reference=w280, error in=w279, "Offset"=w282) -> (error out=w275:errorcluster, "SetVchOffset"=w281:sgl)  [unwired: 1 in, 2 out]
                n707 = local write "Vch Offset"(w281) -> ()
                n708 = Build Array(w289, w288, w275, w287, w286) -> (w290:errorcluster[])
                n709 = Merge Errors(w290) -> (w285:errorcluster)
              }
            }
            n710 = Unbundle By Name(w240) -> ("status"=w241:bool)
            n711 = local write "ForcePstatFunctionUpdate"(FALSE ("ForcePstatFunctionUpdate")) -> ()
            n712 = call "Pstat Settings Error"("Enable"=w241) -> ()  [unwired: 9 in, 2 out]
          }
          event "Cycles", "Signal Type", "Acq. Frequency", "Signal Frequency", "Amplitude", "DC Offset", "Phase Offset", "Initial", "Final", "Scan Rate", "Continuous", "Duty Cycle": Value Change {
            # "Signal Tweak Loop"
            n713 = event-data() -> ("OldVal"=w341:variant, "NewVal"=w340:variant, "CtlRef"=w339:refnum<vi>)  [unwired: 1 in]
            n714 = local read "Continuous"() -> (w342:bool)
            n715 = local read "Signal Type"() -> (w347:u16)
            n716 = local read "Taking Data"() -> (w346:bool)
            n717 = Select(t=2, s=w342, f=0) -> (s? t:f=w343:i32)
            n718 = property on="Cycles" class="DigNum (strict)"("Disabled"=w343) -> ()  [unwired: 2 in, 2 out]
            n719 = stacked-sequence {
              tunnel: w347 -> [w348 w379]
              tunnel: w346 -> [_ w378]
              tunnel: w341 -> [_ w377]
              tunnel: w340 -> [_ w376]
              tunnel: w339 -> [_ w375]
              frame #0 {
                # "Adjust front panel according to signal type"
                n720 = case shown="Default" w348 {
                  frame 0, 1, 4 {
                    w350 = FALSE ("Visible")
                    (unwired) FALSE ("Visible")
                    w352 = TRUE ("Visible")
                    n721 = property on="Signal Frequency" class="DigNum (strict)"("Visible"=w352) -> ()  [unwired: 2 in, 2 out]
                    n722 = property on="Amplitude" class="DigNum (strict)"("Visible"=w352) -> ()  [unwired: 2 in, 2 out]
                    n723 = property on="DC Offset" class="DigNum (strict)"("Visible"=w352) -> ()  [unwired: 2 in, 2 out]
                    n724 = property on="Phase Offset" class="DigNum (strict)"("Visible"=w352) -> ()  [unwired: 2 in, 2 out]
                    n725 = property on="Acq. Frequency" class="DigNum (strict)"("Visible"=w352) -> ()  [unwired: 2 in, 2 out]
                    n726 = property on="Cycles" class="DigNum (strict)"("Visible"=w352) -> ()  [unwired: 2 in, 2 out]
                    n727 = property on="Continuous" class="Bool (strict)"("Visible"=w352) -> ()  [unwired: 2 in, 2 out]
                    n728 = property on="Duty Cycle" class="DigNum (strict)"("Visible"=FALSE) -> ()  [unwired: 2 in, 2 out]
                    n729 = property on="Filename" class="Path"("Visible"=FALSE) -> ()  [unwired: 2 in, 2 out]
                    n730 = property on="Final" class="DigNum (strict)"("Visible"=w350) -> ()  [unwired: 2 in, 2 out]
                    n731 = property on="Initial" class="DigNum (strict)"("Visible"=w350) -> ()  [unwired: 2 in, 2 out]
                    n732 = property on="Scan Rate" class="DigNum (strict)"("Visible"=w350) -> ()  [unwired: 2 in, 2 out]
                  }
                  frame 2 {
                    w354 = TRUE ("Visible")
                    (unwired) FALSE ("Visible")
                    w355 = FALSE ("Visible")
                    # "Triangle"
                    n733 = property on="Signal Frequency" class="DigNum (strict)"("Visible"=w355) -> ()  [unwired: 2 in, 2 out]
                    n734 = property on="Amplitude" class="DigNum (strict)"("Visible"=w355) -> ()  [unwired: 2 in, 2 out]
                    n735 = property on="DC Offset" class="DigNum (strict)"("Visible"=w355) -> ()  [unwired: 2 in, 2 out]
                    n736 = property on="Phase Offset" class="DigNum (strict)"("Visible"=w355) -> ()  [unwired: 2 in, 2 out]
                    n737 = property on="Duty Cycle" class="DigNum (strict)"("Visible"=FALSE) -> ()  [unwired: 2 in, 2 out]
                    n738 = property on="Filename" class="Path"("Visible"=FALSE) -> ()  [unwired: 2 in, 2 out]
                    n739 = property on="Final" class="DigNum (strict)"("Visible"=w354) -> ()  [unwired: 2 in, 2 out]
                    n740 = property on="Initial" class="DigNum (strict)"("Visible"=w354) -> ()  [unwired: 2 in, 2 out]
                    n741 = property on="Scan Rate" class="DigNum (strict)"("Visible"=w354) -> ()  [unwired: 2 in, 2 out]
                    n742 = property on="Acq. Frequency" class="DigNum (strict)"("Visible"=w354) -> ()  [unwired: 2 in, 2 out]
                    n743 = property on="Cycles" class="DigNum (strict)"("Visible"=w354) -> ()  [unwired: 2 in, 2 out]
                    n744 = property on="Continuous" class="Bool (strict)"("Visible"=w354) -> ()  [unwired: 2 in, 2 out]
                  }
                  frame 3 {
                    w359 = FALSE ("Visible")
                    (unwired) FALSE ("Visible")
                    w361 = TRUE ("Visible")
                    n745 = property on="Signal Frequency" class="DigNum (strict)"("Visible"=w361) -> ()  [unwired: 2 in, 2 out]
                    n746 = property on="Amplitude" class="DigNum (strict)"("Visible"=w361) -> ()  [unwired: 2 in, 2 out]
                    n747 = property on="DC Offset" class="DigNum (strict)"("Visible"=w361) -> ()  [unwired: 2 in, 2 out]
                    n748 = property on="Acq. Frequency" class="DigNum (strict)"("Visible"=w361) -> ()  [unwired: 2 in, 2 out]
                    n749 = property on="Cycles" class="DigNum (strict)"("Visible"=w361) -> ()  [unwired: 2 in, 2 out]
                    n750 = property on="Continuous" class="Bool (strict)"("Visible"=w361) -> ()  [unwired: 2 in, 2 out]
                    n751 = property on="Duty Cycle" class="DigNum (strict)"("Visible"=TRUE) -> ()  [unwired: 2 in, 2 out]
                    n752 = property on="Phase Offset" class="DigNum (strict)"("Visible"=FALSE) -> ()  [unwired: 2 in, 2 out]
                    n753 = property on="Filename" class="Path"("Visible"=FALSE) -> ()  [unwired: 2 in, 2 out]
                    n754 = property on="Final" class="DigNum (strict)"("Visible"=w359) -> ()  [unwired: 2 in, 2 out]
                    n755 = property on="Initial" class="DigNum (strict)"("Visible"=w359) -> ()  [unwired: 2 in, 2 out]
                    n756 = property on="Scan Rate" class="DigNum (strict)"("Visible"=w359) -> ()  [unwired: 2 in, 2 out]
                  }
                  frame 5, 6 {
                    w363 = TRUE ("Visible")
                    (unwired) FALSE ("Visible")
                    w364 = FALSE ("Visible")
                    # "Ramp"
                    n757 = property on="Signal Frequency" class="DigNum (strict)"("Visible"=w364) -> ()  [unwired: 2 in, 2 out]
                    n758 = property on="Amplitude" class="DigNum (strict)"("Visible"=w364) -> ()  [unwired: 2 in, 2 out]
                    n759 = property on="DC Offset" class="DigNum (strict)"("Visible"=w364) -> ()  [unwired: 2 in, 2 out]
                    n760 = property on="Phase Offset" class="DigNum (strict)"("Visible"=w364) -> ()  [unwired: 2 in, 2 out]
                    n761 = property on="Cycles" class="DigNum (strict)"("Visible"=w364) -> ()  [unwired: 2 in, 2 out]
                    n762 = property on="Continuous" class="Bool (strict)"("Visible"=w364) -> ()  [unwired: 2 in, 2 out]
                    n763 = property on="Duty Cycle" class="DigNum (strict)"("Visible"=FALSE) -> ()  [unwired: 2 in, 2 out]
                    n764 = property on="Filename" class="Path"("Visible"=FALSE) -> ()  [unwired: 2 in, 2 out]
                    n765 = property on="Final" class="DigNum (strict)"("Visible"=w363) -> ()  [unwired: 2 in, 2 out]
                    n766 = property on="Initial" class="DigNum (strict)"("Visible"=w363) -> ()  [unwired: 2 in, 2 out]
                    n767 = property on="Scan Rate" class="DigNum (strict)"("Visible"=w363) -> ()  [unwired: 2 in, 2 out]
                    n768 = property on="Acq. Frequency" class="DigNum (strict)"("Visible"=w363) -> ()  [unwired: 2 in, 2 out]
                  }
                  frame 7 {
                    w368 = FALSE ("Visible")
                    w366 = TRUE ("Visible")
                    w370 = FALSE ("Visible")
                    # "Single Point"
                    n769 = property on="Signal Frequency" class="DigNum (strict)"("Visible"=w370) -> ()  [unwired: 2 in, 2 out]
                    n770 = property on="Amplitude" class="DigNum (strict)"("Visible"=w370) -> ()  [unwired: 2 in, 2 out]
                    n771 = property on="Phase Offset" class="DigNum (strict)"("Visible"=w370) -> ()  [unwired: 2 in, 2 out]
                    n772 = property on="Cycles" class="DigNum (strict)"("Visible"=w370) -> ()  [unwired: 2 in, 2 out]
                    n773 = property on="Continuous" class="Bool (strict)"("Visible"=w370) -> ()  [unwired: 2 in, 2 out]
                    n774 = property on="Acq. Frequency" class="DigNum (strict)"("Visible"=w366) -> ()  [unwired: 2 in, 2 out]
                    n775 = property on="DC Offset" class="DigNum (strict)"("Visible"=w366) -> ()  [unwired: 2 in, 2 out]
                    n776 = property on="Duty Cycle" class="DigNum (strict)"("Visible"=FALSE) -> ()  [unwired: 2 in, 2 out]
                    n777 = property on="Filename" class="Path"("Visible"=FALSE) -> ()  [unwired: 2 in, 2 out]
                    n778 = property on="Final" class="DigNum (strict)"("Visible"=w368) -> ()  [unwired: 2 in, 2 out]
                    n779 = property on="Initial" class="DigNum (strict)"("Visible"=w368) -> ()  [unwired: 2 in, 2 out]
                    n780 = property on="Scan Rate" class="DigNum (strict)"("Visible"=w368) -> ()  [unwired: 2 in, 2 out]
                  }
                  frame 8 {
                    w372 = FALSE ("Visible")
                    w373 = TRUE ("Visible")
                    (unwired) FALSE ("Visible")
                    w374 = FALSE ("Visible")
                    # "From File"
                    n781 = property on="Signal Frequency" class="DigNum (strict)"("Visible"=w374) -> ()  [unwired: 2 in, 2 out]
                    n782 = property on="Amplitude" class="DigNum (strict)"("Visible"=w374) -> ()  [unwired: 2 in, 2 out]
                    n783 = property on="DC Offset" class="DigNum (strict)"("Visible"=w374) -> ()  [unwired: 2 in, 2 out]
                    n784 = property on="Phase Offset" class="DigNum (strict)"("Visible"=w374) -> ()  [unwired: 2 in, 2 out]
                    n785 = property on="Duty Cycle" class="DigNum (strict)"("Visible"=FALSE) -> ()  [unwired: 2 in, 2 out]
                    n786 = property on="Filename" class="Path"("Visible"=w373) -> ()  [unwired: 2 in, 2 out]
                    n787 = property on="Acq. Frequency" class="DigNum (strict)"("Visible"=w373) -> ()  [unwired: 2 in, 2 out]
                    n788 = property on="Cycles" class="DigNum (strict)"("Visible"=w373) -> ()  [unwired: 2 in, 2 out]
                    n789 = property on="Continuous" class="Bool (strict)"("Visible"=w373) -> ()  [unwired: 2 in, 2 out]
                    n790 = property on="Scan Rate" class="DigNum (strict)"("Visible"=w372) -> ()  [unwired: 2 in, 2 out]
                    n791 = property on="Final" class="DigNum (strict)"("Visible"=w372) -> ()  [unwired: 2 in, 2 out]
                    n792 = property on="Initial" class="DigNum (strict)"("Visible"=w372) -> ()  [unwired: 2 in, 2 out]
                  }
                  frame Default {
                  }
                }
              }
              frame #1 {
                n793 = case shown="True" w378 {
                  tunnel: w379 -> [_ w387]
                  tunnel: w377 -> [_ w382]
                  tunnel: w376 -> [_ w380]
                  tunnel: w375 -> [_ w381]
                  frame False {
                  }
                  frame True {
                    # "Nyquist Criterion"
                    n794 = local read "Signal Frequency"() -> (w383:dbl)
                    n795 = local read "Acq. Frequency"() -> (w384:dbl)
                    n796 = local read "Signal Type"() -> (w386:u16)
                    n797 = case shown="0, 1, 3, 4" w386 {
                      tunnel: w384 -> [_ w393]
                      tunnel: w383 -> [_ w391]
                      tunnel: [TRUE w389] -> w385
                      frame Default {
                      }
                      frame 0, 1, 3, 4 {
                        n798 = Multiply(x=2.0, y=w391) -> (x*y=w392:dbl)
                        n799 = Greater?(x=w393, y=w392) -> (0:w389:bool)
                      }
                    }
                    n800 = case shown="True" w385 {
                      tunnel: w383 -> [_ w417]
                      tunnel: w384 -> [_ w416]
                      tunnel: w387 -> [_ w413]
                      tunnel: w382 -> [_ w406]
                      tunnel: w380 -> [_ w405]
                      tunnel: w381 -> [_ w402]
                      frame False {
                        n801 = call "Nyquist Criterion"("Enable"=TRUE) -> ()  [unwired: 9 in, 2 out]
                      }
                      frame True {
                        w396 = 0 items=["SigTweakStyleReset", "SigTweakStyleContinue", "SigTweakStyleScale"] ("Tweak Style")
                        # "Check to see if the signal type changed,\nIf so, we want to RESET the tweak rather\nthan try and transition gracefully."
                        n802 = local read "Amplitude"() -> (w418:dbl)
                        n803 = local read "Continuous"() -> (w414:bool)
                        n804 = local read "Cycles"() -> (w415:u32)
                        n805 = local read "Phase Offset"() -> (w420:dbl)
                        n806 = local read "Duty Cycle"() -> (w425:dbl)
                        n807 = local read "DC Offset"() -> (w419:dbl)
                        n808 = local read "Scan Rate"() -> (w421:dbl)
                        n809 = local read "Final"() -> (w422:dbl)
                        n810 = local read "Initial"() -> (w423:dbl)
                        n811 = Not Equal?(x=w406, y=w405) -> (x != y?=w400:bool)
                        n812 = case shown="5, 6" w413 {
                          selector: w413 -> [w437 w453 w480 w495 _ _ _]
                          tunnel: w414 -> [w439 w455 w482 _ _ w528 w544]
                          tunnel: w415 -> [w438 w454 w481 _ _ w527 w543]
                          tunnel: w416 -> [w436 w452 w479 w503 w519 w526 w549]
                          tunnel: w417 -> [w428 _ w470 _ _ _ _]
                          tunnel: w418 -> [w435 _ w478 _ _ _ _]
                          tunnel: w419 -> [w434 _ w477 _ w513 _ _]
                          tunnel: w420 -> [w433 _ w476 _ _ _ _]
                          tunnel: w421 -> [_ w451 _ w502 _ _ _]
                          tunnel: w422 -> [_ w450 _ w501 _ _ _]
                          tunnel: w423 -> [_ w449 _ w500 _ _ _]
                          tunnel: [w432 w447 w475 w497 w517 w523 dbl[] []] -> w411
                          tunnel: [w431 w448 w474 1 ("t") -1 ("t") w524 w542] -> w412
                          tunnel: [w430 w446 w473 w498 w516 w525 w548] -> w408
                          tunnel: [w429 w445 w472 w496 0 ("error") 0 ("error") 0 ("error")] -> w424
                          tunnel: w425 -> [_ _ w471 _ _ _ _]
                          tunnel: [w426 w442 w468 w485 w514 w521 w541] -> w397
                          tunnel: w402 -> [_ _ _ w486 _ _ _]
                          frame 0, 1, 4 {
                            w426 = 2 items=["SigTweakStyleReset", "SigTweakStyleContinue", "SigTweakStyleScale"] ("Tweak Style")
                            # "Sine, Cosine, Sawtooth"
                            n813 = Select(t=-1, s=w439, f=w438) -> (s? t:f=w431:u32)
                            n814 = Reciprocal(x=w428) -> (1/x=w427:dbl)
                            n815 = Reciprocal(x=w436) -> (1/x=w430:dbl)
                            n816 = Multiply(x=w436, y=w427) -> (x*y=w441:dbl)
                            n817 = call <vilib>:"Signal Generator by Duration.vi"("signal type"=w437, "duration"=w427, "# of samples"=w441, "frequency"=w428, "amplitude"=w435, "dc offset"=w434, "phase in"=w433) -> ("signal"=w432:dbl[], "error"=w429:i32)  [unwired: 5 in, 2 out]
                          }
                          frame 2 {
                            w442 = 0 items=["SigTweakStyleReset", "SigTweakStyleContinue", "SigTweakStyleScale"] ("Tweak Style")
                            # "Triangle"
                            n818 = Select(t=-1, s=w455, f=w454) -> (s? t:f=w448:u32)
                            n819 = Subtract(x=w450, y=w449) -> (x-y=w460:dbl)
                            n820 = Add(x=w450, y=w449) -> (x+y=w456:dbl)
                            n821 = Divide(x=w460, y=w451) -> (x/y=w465:dbl)
                            n822 = Divide(x=w460, y=2.0) -> (x/y=w459:dbl)
                            n823 = Divide(x=w456, y=2.0) -> (x/y=w458:dbl)
                            n824 = Reciprocal(x=w452) -> (1/x=w446:dbl)
                            n825 = Absolute Value(x=w465) -> (abs(x)=w464:dbl)
                            n826 = Multiply(x=w464, y=2.0) -> (x*y=w443:dbl)
                            n827 = Reciprocal(x=w443) -> (1/x=w444:dbl)
                            n828 = Multiply(x=w452, y=w443) -> (x*y=w467:dbl)
                            n829 = call <vilib>:"Signal Generator by Duration.vi"("signal type"=w453, "duration"=w443, "# of samples"=w467, "frequency"=w444, "amplitude"=w459, "dc offset"=w458, "phase in"=270.0) -> ("signal"=w447:dbl[], "error"=w445:i32)  [unwired: 5 in, 2 out]
                          }
                          frame 3 {
                            w468 = 2 items=["SigTweakStyleReset", "SigTweakStyleContinue", "SigTweakStyleScale"] ("Tweak Style")
                            # "Square Wave"
                            n830 = Select(t=-1, s=w482, f=w481) -> (s? t:f=w474:u32)
                            n831 = Reciprocal(x=w470) -> (1/x=w469:dbl)
                            n832 = Reciprocal(x=w479) -> (1/x=w473:dbl)
                            n833 = Multiply(x=w479, y=w469) -> (x*y=w484:dbl)
                            n834 = call <vilib>:"Signal Generator by Duration.vi"("signal type"=w480, "duration"=w469, "# of samples"=w484, "frequency"=w470, "amplitude"=w478, "dc offset"=w477, "phase in"=w476, "square wave duty cycle (%)"=w471) -> ("signal"=w475:dbl[], "error"=w472:i32)  [unwired: 4 in, 2 out]
                          }
                          frame 5, 6 {
                            # "Ramp"
                            n835 = control-ref of="Initial"() -> (w490:refnum<vi>)
                            n836 = control-ref of="Scan Rate"() -> (w487:refnum<vi>)
                            n837 = Subtract(x=w501, y=w500) -> (x-y=w505:dbl)
                            n838 = Divide(x=w505, y=w502) -> (x/y=w504:dbl)
                            n839 = To More Generic Class(target class=w486, reference=w490) -> (generic class reference=w489:refnum<vi>)
                            n840 = To More Generic Class(target class=w486, reference=w487) -> (generic class reference=w488:refnum<vi>)
                            n841 = Absolute Value(x=w504) -> (abs(x)=w493:dbl)
                            n842 = Equal?(x=w486, y=w489) -> (x = y?=w491:bool)
                            n843 = Equal?(x=w486, y=w488) -> (x = y?=w492:bool)
                            n844 = Reciprocal(x=w503) -> (1/x=w498:dbl)
                            n845 = Reciprocal(x=w493) -> (1/x=w494:dbl)
                            n846 = case shown="False" w491 {
                              tunnel: w492 -> [w509 _]
                              tunnel: [w508 w512] -> w485
                              frame False {
                                n847 = case shown="False" w509 {
                                tunnel: [w510 w511] -> w508
                                frame False {
                                w510 = 1 items=["SigTweakStyleReset", "SigTweakStyleContinue", "SigTweakStyleScale"] ("Tweak Style")
                                }
                                frame True {
                                w511 = 2 items=["SigTweakStyleReset", "SigTweakStyleContinue", "SigTweakStyleScale"] ("Tweak Style")
                                }
                                }
                              }
                              frame True {
                                w512 = 0 items=["SigTweakStyleReset", "SigTweakStyleContinue", "SigTweakStyleScale"] ("Tweak Style")
                              }
                            }
                            n848 = Multiply(x=w503, y=w493) -> (x*y=w507:dbl)
                            n849 = call <vilib>:"Signal Generator by Duration.vi"("signal type"=w495, "duration"=w493, "# of samples"=w507, "frequency"=w494, "amplitude"=w505, "dc offset"=w500, "phase in"=0.0) -> ("signal"=w497:dbl[], "error"=w496:i32)  [unwired: 5 in, 2 out]
                          }
                          frame 7 {
                            w514 = 0 items=["SigTweakStyleReset", "SigTweakStyleContinue", "SigTweakStyleScale"] ("Tweak Style")
                            # "Single Point"
                            n850 = Reciprocal(x=w519) -> (1/x=w516:dbl)
                            n851 = Initialize Array(w513, 1 ("dimension size")) -> (w517:dbl[])
                          }
                          frame 8 {
                            w521 = 0 items=["SigTweakStyleReset", "SigTweakStyleContinue", "SigTweakStyleScale"] ("Tweak Style")
                            (unwired) TRUE ("convert eol (F)")
                            # "From File"
                            n852 = local read "Filename"() -> (w539:path)
                            n853 = call <vilib>:"Open_Create_Replace File.vi"("file path"=w539) -> ("error out"=w536:errorcluster, "file size (bytes)"=w537:i32, "new file path"=w538:path, "refnum"=w540:refnum<file>)  [unwired: 7 in]
                            n854 = local write "Filename"(w538) -> ()
                            n855 = Select(t=-1, s=w528, f=w527) -> (s? t:f=w524:u32)
                            n856 = Reciprocal(x=w526) -> (1/x=w525:dbl)
                            n857 = Read from Text File(file (use dialog)=w540, count=w537, error in=w536) -> (refnum out=w529:refnum<file>, text=w531:string, error out=w530:errorcluster)  [unwired: 1 in, 1 out]
                            n858 = local write "From File Refnum"(w529) -> ()
                            n859 = Close File(refnum=w529, error in=w530) -> ()  [unwired: 2 out]
                            n860 = local write "File Data"(w531) -> ()
                            n861 = Spreadsheet String To Array(delimiter (Tab)="\n", format string="%f", spreadsheet string=w531, array type (2D Dbl)=dbl[] [] ("initialized array")) -> (array=w523:dbl[])
                          }
                          frame Default {
                            w541 = 0 items=["SigTweakStyleReset", "SigTweakStyleContinue", "SigTweakStyleScale"] ("Tweak Style")
                            n862 = Reciprocal(x=w549) -> (1/x=w548:dbl)
                            n863 = Select(t=-1, s=w544, f=w543) -> (s? t:f=w542:u32)
                          }
                        }
                        n864 = call <vilib>:"Error Cluster From Error Code.vi"("error code (0)"=w424) -> ("error out"=w395:errorcluster)  [unwired: 8 in]
                        n865 = control-ref of="Signal Type"() -> (w404:refnum<vi>)
                        n866 = To More Generic Class(target class=w402, reference=w404) -> (generic class reference=w403:refnum<vi>)
                        n867 = property class="WFChart (strict)"("X Scale.Offset and Multiplier:Multiplier"=w408) -> ()  [unwired: 2 in, 2 out]
                        n868 = Equal?(x=w402, y=w403) -> (x = y?=w399:bool)
                        n869 = And(x=w400, y=w399) -> (x .and. y?=w398:bool)
                        n870 = local read "Signal"() -> (w407:refnum<k7>)
                        n871 = Select(t=w396, s=w398, f=w397) -> (s? t:f=w401:i32)
                        n872 = call "SigArrayTweak.vi"("Signal IN"=w407, "Style"=w401, "Cycles"=w412, "Sample Rate"=w408, "Signal Array"=w411, "error in"=w395) -> ("error out"=w410:errorcluster)  [unwired: 8 in, 1 out]
                        n873 = Unbundle By Name(w410) -> ("status"=w409:bool)
                        n874 = call "Tweak Error"("Enable"=w409) -> ()  [unwired: 9 in, 2 out]
                      }
                    }
                  }
                }
              }
            }
          }
          event "Device List Change": Value Change {
            w561 = T14 0 items=["no dialog", "OK message", "continue or stop message", "OK message + warnings", "continue/stop + warnings"] ("type of dialog (OK msg:1)")
            n875 = event-data() -> ("CtlRef"=w551:refnum<vi>)  [unwired: 1 in, 5 out]
            n876 = property class="Bool (strict)"(reference=w551, "Value"=FALSE ("Device List Change")) -> ()  [unwired: 1 in, 2 out]
            n877 = local read "Device List"() -> (w560:refnum<k7>)
            n878 = local read "Section List"() -> (w558:string[])
            n879 = local read "Device"() -> (w559:u16)
            n880 = call "UpdateDeviceList.vi"("Section List"=w558, "Device"=w559, "Device List"=w560) -> ("error out"=w553:errorcluster, "New Section List"=w557:string[], "New Label List"=w555:string[], "New Device Index"=w554:i32)  [unwired: 5 in]
            n881 = local write "Index of Device (Device Change)"(w554) -> ()
            n882 = local write "Section List"(w557) -> ()
            n883 = Not Equal?(x=w554, y=-1) -> (x != y?=w564:bool)
            n884 = local read "Taking Data"() -> (w569:bool)
            n885 = Select(t=w554, s=w564, f=0) -> (s? t:f=w565:i32)
            n886 = Not(x=w564) -> (.not. x?=w563:bool)
            n887 = property on="Device" class="Ring (strict)"(error in=w553, "Strings []"=w555, "Value (Signaling)"=w565) -> (error out=w556:errorcluster)  [unwired: 1 in, 1 out]
            n888 = And(x=w563, y=w569) -> (x .and. y?=w568:bool)
            n889 = case shown="True" w568 {
              tunnel: w556 -> [w580 w582]
              tunnel: [w580 w582] -> w562
              frame False {
              }
              frame True {
                # "Stop and notify User"
                n890 = local write "Start/Stop"(FALSE ("Start/Stop")) -> ()
                n891 = local write "Device Open"(FALSE ("Device Gone")) -> ()
                n892 = local write "Device Gone"(TRUE ("Device Gone")) -> ()
              }
            }
            n893 = local read "[user-defined descriptions]"() -> (w571:string[])
            n894 = local read "[user-defined codes]"() -> (w570:u32[])
            n895 = local read "Taking Data"() -> (w552:bool)
            n896 = call <vilib>:"General Error Handler.vi"("[user-defined codes]"=w570, "[user-defined descriptions]"=w571, "type of dialog (OK msg:1)"=w561, "error in (no error)"=w562) -> ("error out"=w572:errorcluster)  [unwired: 7 in, 4 out]
            n897 = case shown="True" w552 {
              tunnel: w572 -> [w573 w577]
              frame False {
                n898 = case shown="Error" w573 {
                  frame No Error {
                    w574 = u8 0 ("Disabled")
                    # "Enable appropriate menu stuff"
                    n899 = property on="Start/Stop" class="Bool (strict)"("Disabled"=w574) -> ()  [unwired: 2 in, 2 out]
                    n900 = property on="Signal Type" class="Ring (strict)"("Disabled"=w574) -> ()  [unwired: 2 in, 2 out]
                    n901 = property on="Device" class="Ring (strict)"("Disabled"=w574) -> ()  [unwired: 2 in, 2 out]
                    n902 = property on="CtrlMode" class="Ring (strict)"("Disabled"=w574) -> ()  [unwired: 2 in, 2 out]
                    n903 = property on="I/E Range" class="Ring (strict)"("Disabled"=w574) -> ()  [unwired: 2 in, 2 out]
                    n904 = property on="Vch Range" class="Ring (strict)"("Disabled"=w574) -> ()  [unwired: 2 in, 2 out]
                    n905 = property on="Ich Range" class="Ring (strict)"("Disabled"=w574) -> ()  [unwired: 2 in, 2 out]
                    n906 = property on="Vch Filter" class="Ring (strict)"("Disabled"=w574) -> ()  [unwired: 2 in, 2 out]
                    n907 = property on="Ich Filter" class="Ring (strict)"("Disabled"=w574) -> ()  [unwired: 2 in, 2 out]
                    n908 = property on="Vch Offset" class="DigNum (strict)"("Disabled"=w574) -> ()  [unwired: 2 in, 2 out]
                    n909 = property on="Ich Offset" class="DigNum (strict)"("Disabled"=w574) -> ()  [unwired: 2 in, 2 out]
                    n910 = property on="I/E Stability" class="Ring (strict)"("Disabled"=w574) -> ()  [unwired: 2 in, 2 out]
                    n911 = property on="CA Speed" class="Ring (strict)"("Disabled"=w574) -> ()  [unwired: 2 in, 2 out]
                  }
                  frame Error {
                    w576 = u16 0 items=[""] ("Device")
                    w575 = u8 2 ("Disabled")
                    # "Disable appropriate menu stuff"
                    n912 = property on="Start/Stop" class="Bool (strict)"("Disabled"=w575) -> ()  [unwired: 2 in, 2 out]
                    n913 = property on="CtrlMode" class="Ring (strict)"("Disabled"=w575) -> ()  [unwired: 2 in, 2 out]
                    n914 = property on="Device" class="Ring (strict)"("Disabled"=w575, "Value"=w576) -> ()  [unwired: 2 in, 2 out]
                    n915 = property on="I/E Range" class="Ring (strict)"("Disabled"=w575, "Value"=w576) -> ()  [unwired: 2 in, 2 out]
                    n916 = property on="Vch Range" class="Ring (strict)"("Disabled"=w575, "Value"=w576) -> ()  [unwired: 2 in, 2 out]
                    n917 = property on="Ich Range" class="Ring (strict)"("Disabled"=w575, "Value"=w576) -> ()  [unwired: 2 in, 2 out]
                    n918 = property on="Vch Filter" class="Ring (strict)"("Disabled"=w575, "Value"=w576) -> ()  [unwired: 2 in, 2 out]
                    n919 = property on="Ich Filter" class="Ring (strict)"("Disabled"=w575, "Value"=w576) -> ()  [unwired: 2 in, 2 out]
                    n920 = property on="Vch Offset" class="DigNum (strict)"("Disabled"=w575) -> ()  [unwired: 2 in, 2 out]
                    n921 = property on="Ich Offset" class="DigNum (strict)"("Disabled"=w575) -> ()  [unwired: 2 in, 2 out]
                    n922 = property on="I/E Stability" class="Ring (strict)"("Disabled"=w575) -> ()  [unwired: 2 in, 2 out]
                    n923 = property on="CA Speed" class="Ring (strict)"("Disabled"=w575) -> ()  [unwired: 2 in, 2 out]
                  }
                }
              }
              frame True {
                n924 = case shown="Error" w577 {
                  frame No Error {
                  }
                  frame Error {
                    w579 = u16 0 items=[""] ("Device")
                    w578 = u8 2 ("Disabled")
                    # "Disable appropriate menu stuff"
                    n925 = property on="Start/Stop" class="Bool (strict)"("Disabled"=w578) -> ()  [unwired: 2 in, 2 out]
                    n926 = property on="CtrlMode" class="Ring (strict)"("Disabled"=w578) -> ()  [unwired: 2 in, 2 out]
                    n927 = property on="Device" class="Ring (strict)"("Disabled"=w578, "Value"=w579) -> ()  [unwired: 2 in, 2 out]
                    n928 = property on="I/E Range" class="Ring (strict)"("Disabled"=w578, "Value"=w579) -> ()  [unwired: 2 in, 2 out]
                    n929 = property on="Vch Range" class="Ring (strict)"("Disabled"=w578, "Value"=w579) -> ()  [unwired: 2 in, 2 out]
                    n930 = property on="Ich Range" class="Ring (strict)"("Disabled"=w578, "Value"=w579) -> ()  [unwired: 2 in, 2 out]
                    n931 = property on="Vch Filter" class="Ring (strict)"("Disabled"=w578, "Value"=w579) -> ()  [unwired: 2 in, 2 out]
                    n932 = property on="Ich Filter" class="Ring (strict)"("Disabled"=w578, "Value"=w579) -> ()  [unwired: 2 in, 2 out]
                    n933 = property on="Vch Offset" class="DigNum (strict)"("Disabled"=w578) -> ()  [unwired: 2 in, 2 out]
                    n934 = property on="Ich Offset" class="DigNum (strict)"("Disabled"=w578) -> ()  [unwired: 2 in, 2 out]
                    n935 = property on="I/E Stability" class="Ring (strict)"("Disabled"=w578) -> ()  [unwired: 2 in, 2 out]
                    n936 = property on="CA Speed" class="Ring (strict)"("Disabled"=w578) -> ()  [unwired: 2 in, 2 out]
                  }
                }
              }
            }
          }
          event "Device": Value Change {
            n937 = event-data() -> ("NewVal"=w586:u16)  [unwired: 1 in, 5 out]
            n938 = local read "Section List"() -> (w587:string[])
            n939 = Index Array(array=w587, index=w586) -> (element=w585:string)
            n940 = property on="Section" class="Str"("Value (Signaling)"=w585) -> ()  [unwired: 2 in, 2 out]
          }
          event "Section": Value Change {
            n941 = event-data() -> ("OldVal"=w589:string, "NewVal"=w588:string)  [unwired: 1 in, 4 out]
            n942 = Not Equal?(x=w589, y=w588) -> (x != y?=w590:bool)
            n943 = case shown="True" w590 {
              tunnel: w588 -> [_ w597]
              frame False {
              }
              frame True {
                n944 = local read "Device Open"() -> (w602:bool)
                n945 = local read "Pstat"() -> (w604:refnum<k7>)
                n946 = case shown="True" w602 {
                  tunnel: w604 -> [w649 w653]
                  tunnel: [w649 w652] -> w603
                  tunnel: [errorcluster {"status"=FALSE, "code"=0, "source"=""} ("error out") w650] -> w601
                  frame False {
                  }
                  frame True {
                    n947 = invoke class="IGamryPstat" method="Close"(reference=w653, "Safe"=TRUE) -> (reference out=w652:refnum<k7>, error out=w650:errorcluster)  [unwired: 2 in, 2 out]
                  }
                }
                n948 = invoke class="IGamryPstat" method="Init"(reference=w603, error in=w601, "Section"=w597) -> (reference out=w600:refnum<k7>, error out=w599:errorcluster)  [unwired: 1 in, 2 out]
                n949 = invoke class="IGamryPstat" method="Open"(reference=w600, error in=w599) -> (reference out=w593:refnum<k7>, error out=w598:errorcluster)  [unwired: 1 in, 1 out]
                n950 = case shown="No Error" w598 {
                  selector: w598 -> [w644 w646]
                  tunnel: [w644 w646] -> w594
                  frame No Error {
                    n951 = local write "Device Open"(TRUE ("Device Open")) -> ()
                  }
                  frame Error {
                    n952 = local write "Device Open"(FALSE ("Device Open")) -> ()
                  }
                }
                n953 = call "HardwareRangeStrings.vi"("error in (no error)"=w594, "Pstat IN"=w593) -> ("error out"=w595:errorcluster, "Hardware Strings"=w591:T8, "Pstat OUT"=w592:refnum<k7>)  [unwired: 7 in]
                n954 = Unbundle By Name(w591) -> ("I/E Ranges"=w636:string[], "First I/E Range"=w624:i32, "VchRanges"=w638:string[], "IchRanges"=w637:string[], "VchFilters"=w635:string[], "IchFilters"=w634:string[], "Family"=w596:string, "CA Speeds"=w627:string[])  [unwired: 2 out]
                n955 = invoke class="IGamryPstat" method="CtrlMode"(reference=w592, error in=w595) -> (reference out=w630:refnum<k7>, error out=w631:errorcluster, "CtrlMode"=w639:i32)  [unwired: 1 in]
                n956 = local write "CtrlMode"(w639) -> ()
                n957 = invoke class="IGamryPstat" method="IchRange"(reference=w630, error in=w631) -> (reference out=w628:refnum<k7>, error out=w629:errorcluster, "IchRange"=w641:i32)  [unwired: 1 in]
                n958 = local write "Family"(w596) -> ()
                n959 = local write "Ich Range"(w641) -> ()
                n960 = property on="I/E Range" class="Ring (strict)"("Strings []"=w636) -> ()  [unwired: 2 in, 2 out]
                n961 = property on="Vch Range" class="Ring (strict)"("Strings []"=w638) -> ()  [unwired: 2 in, 2 out]
                n962 = property on="Ich Range" class="Ring (strict)"("Strings []"=w637) -> ()  [unwired: 2 in, 2 out]
                n963 = property on="Vch Filter" class="Ring (strict)"("Strings []"=w635) -> ()  [unwired: 2 in, 2 out]
                n964 = property on="Ich Filter" class="Ring (strict)"("Strings []"=w634) -> ()  [unwired: 2 in, 2 out]
                n965 = property on="CA Speed" class="Ring (strict)"("Strings []"=w627) -> ()  [unwired: 2 in, 2 out]
                n966 = invoke class="IGamryPstat" method="VchRange"(reference=w628, error in=w629) -> (reference out=w611:refnum<k7>, error out=w612:errorcluster, "VchRange"=w640:i32)  [unwired: 1 in]
                n967 = invoke class="IGamryPstat" method="IchFilter"(reference=w611, error in=w612) -> (reference out=w617:refnum<k7>, error out=w618:errorcluster, "IchFilter"=w616:i32)  [unwired: 1 in]
                n968 = local write "Ich Filter"(w616) -> ()
                n969 = invoke class="IGamryPstat" method="VchFilter"(reference=w617, error in=w618) -> (reference out=w609:refnum<k7>, error out=w610:errorcluster, "VchFilter"=w615:i32)  [unwired: 1 in]
                n970 = invoke class="IGamryPstat" method="IchOffset"(reference=w609, error in=w610) -> (reference out=w620:refnum<k7>, error out=w619:errorcluster, "IchOffset"=w614:sgl)  [unwired: 1 in]
                n971 = local write "Ich Offset"(w614) -> ()
                n972 = invoke class="IGamryPstat" method="VchOffset"(reference=w620, error in=w619) -> (reference out=w607:refnum<k7>, error out=w608:errorcluster, "VchOffset"=w613:sgl)  [unwired: 1 in]
                n973 = invoke class="IGamryPstat" method="CASpeed"(reference=w607, error in=w608) -> (reference out=w626:refnum<k7>, error out=w625:errorcluster, "CASpeed"=w622:i32)  [unwired: 1 in]
                n974 = local write "CA Speed"(w622) -> ()
                n975 = invoke class="IGamryPstat" method="IEStability"(reference=w626, error in=w625) -> (reference out=w605:refnum<k7>, error out=w606:errorcluster, "IEStability"=w623:i32)  [unwired: 1 in]
                n976 = local write "I/E Stability"(w623) -> ()
                n977 = local write "Vch Range"(w640) -> ()
                n978 = local write "Vch Filter"(w615) -> ()
                n979 = local write "Vch Offset"(w613) -> ()
                n980 = invoke class="IGamryPstat" method="IERange"(reference=w605, error in=w606) -> (error out=w621:errorcluster, "IERange"=w642:i32)  [unwired: 1 in, 1 out]
                n981 = local read "[user-defined descriptions]"() -> (w632:string[])
                n982 = local read "[user-defined codes]"() -> (w633:u32[])
                n983 = Subtract(x=w642, y=w624) -> (x-y=w643:i32)
                n984 = local write "I/E Range"(w643) -> ()
                n985 = local write "First I/E Range"(w624) -> ()
                n986 = call <vilib>:"General Error Handler.vi"("[user-defined codes]"=w633, "[user-defined descriptions]"=w632, "error in (no error)"=w621) -> ()  [unwired: 8 in, 5 out]
              }
            }
          }
        }
        n987 = local read "Close"() -> (w165:bool)
        n988 = Not(x=w165) -> (.not. x?=w164:bool)
      }
    }
    frame #3 {
      w1233 = 0.0
      w1230 = u8 0 ("Disabled")
      w1231 = u16 0 items=[""] ("I/E Range")
      w1238 = 0 ("First I/E Range")
      w1232 = string[] [] ("Strings []")
      w1236 = FALSE ("Begin")
      # "Reset Buttons and Variables"
      n989 = local write "Cell State"(w1236) -> ()
      n990 = local write "Vch Autorange"(w1236) -> ()
      n991 = local write "Ich Autorange"(w1236) -> ()
      n992 = local write "VchOffsetEnable"(w1236) -> ()
      n993 = local write "Device List Change"(w1236) -> ()
      n994 = local write "I/E Autorange"(w1236) -> ()
      n995 = local write "IchOffsetEnable"(w1236) -> ()
      n996 = local write "Start/Stop"(w1236) -> ()
      n997 = local write "Close"(w1236) -> ()
      n998 = local write "Section"("" ("Section")) -> ()
      n999 = property on="Ich Offset" class="DigNum (strict)"("Value"=w1233, "Disabled"=w1230) -> ()  [unwired: 2 in, 2 out]
      n1000 = property on="Device" class="Ring (strict)"("Strings []"=w1232, "Value"=w1231, "Disabled"=w1230) -> ()  [unwired: 2 in, 2 out]
      n1001 = property on="CtrlMode" class="Ring (strict)"("Value"=w1231, "Disabled"=w1230) -> ()  [unwired: 2 in, 2 out]
      n1002 = property on="Vch Offset" class="DigNum (strict)"("Value"=w1233, "Disabled"=w1230) -> ()  [unwired: 2 in, 2 out]
      n1003 = property on="I/E Range" class="Ring (strict)"("Strings []"=w1232, "Value"=w1231, "Disabled"=w1230) -> ()  [unwired: 2 in, 2 out]
      n1004 = property on="CA Speed" class="Ring (strict)"("Strings []"=w1232, "Value"=w1231, "Disabled"=w1230) -> ()  [unwired: 2 in, 2 out]
      n1005 = property on="Ich Filter" class="Ring (strict)"("Strings []"=w1232, "Value"=w1231, "Disabled"=w1230) -> ()  [unwired: 2 in, 2 out]
      n1006 = property on="I/E Range" class="Ring (strict)"("Strings []"=w1232, "Value"=w1231, "Disabled"=w1230) -> ()  [unwired: 2 in, 2 out]
      n1007 = property on="Vch Range" class="Ring (strict)"("Strings []"=w1232, "Value"=w1231, "Disabled"=w1230) -> ()  [unwired: 2 in, 2 out]
      n1008 = property on="Ich Range" class="Ring (strict)"("Strings []"=w1232, "Value"=w1231, "Disabled"=w1230) -> ()  [unwired: 2 in, 2 out]
      n1009 = property on="Vch Filter" class="Ring (strict)"("Strings []"=w1232, "Value"=w1231, "Disabled"=w1230) -> ()  [unwired: 2 in, 2 out]
      n1010 = property on="I/E Autorange" class="Bool (strict)"("Disabled"=w1230) -> ()  [unwired: 2 in, 2 out]
      n1011 = local write "First I/E Range"(w1238) -> ()
      n1012 = local write "Device"(w1238) -> ()
      n1013 = local read "Device List Change Callback"() -> (w1235:refnum<k27>)
      n1014 = Not A Number/Path/Refnum?(number/path/refnum=w1235) -> (NaN/Path/Refnum?=w1234:bool)
      n1015 = case shown="False" w1234 {
        tunnel: w1235 -> [w1239 _]
        frame False {
          n1016 = Unregister For Events(event registration refnum=w1239) -> ()  [unwired: 1 in, 1 out]
        }
        frame True {
        }
      }
    }
  }
  n1017 = while {
    stop <- w1243 continue-if-true
    n1018 = local read "milliseconds to wait"() -> (w1240:u32)
    n1019 = Current VI's Menubar() -> (w1241:refnum<k9>)
    n1020 = local read "Close"() -> (w1244:bool)
    n1021 = Get Menu Selection(0:w1241) -> (6:w1242:string)  [unwired: 3 in, 4 out]
    n1022 = Wait (ms)(milliseconds to wait=w1240) -> ()  [unwired: 1 out]
    n1023 = Not(x=w1244) -> (.not. x?=w1243:bool)
    n1024 = case shown="\"False\", Default" w1242 {
      frame "False", Default {
      }
      frame "MENU_About_VFP" {
        n1025 = local read "Version"() -> (w1245:string)
        n1026 = Concatenate Strings("Virtual Front Panel\nVersion " ("message"), w1245, "\nCopyright 2010\nGamry Instruments, Inc." ("message")) -> (w1248:string)
        n1027 = One Button Dialog(message=w1248) -> ()  [unwired: 1 in, 1 out]
      }
      frame "MENU_Help" {
        w1249 = T14 1 items=["no dialog", "OK message", "continue or stop message", "OK message + warnings", "continue/stop + warnings"] ("type of dialog (OK msg:1)")
        n1028 = property class="App"() -> ("Application:Kind"=w1251:T13, "Application:Directory Path"=w1250:path)  [unwired: 2 in, 2 out]
        n1029 = case shown="\"Development System\"" w1251 {
          tunnel: [w1256 w1258] -> w1255
          tunnel: w1250 -> [_ w1258]
          frame "Development System" {
            n1030 = Current VI's Path() -> (path=w1257:path)
            n1031 = Strip Path(path=w1257) -> (stripped path=w1256:path)  [unwired: 1 out]
          }
          frame "Run Time System", Default {
          }
        }
        n1032 = Build Path(base path=w1255, name or relative path="VFP600 Manual.pdf") -> (appended path=w1253:path)
        n1033 = call <vilib>:"Open Acrobat Document.vi"("acrobat document"=w1253) -> ("error out"=w1252:errorcluster)  [unwired: 6 in]
        n1034 = call <vilib>:"Simple Error Handler.vi"("type of dialog (OK msg:1)"=w1249, "error in (no error)"=w1252) -> ()  [unwired: 3 in, 5 out]
      }
    }
    n1035 = event shown="[2] Timeout" {
      selector: _ -> [_ _ _]
      dyn-events: _ -> [_ _ _]
      timeout: w1240 -> [_ _ _]
      event Application Instance Close? {
        # "This event is duplicated in Panel Close?"
        n1036 = event-data() -> ()  [unwired: 1 in, 5 out]
        n1037 = local read "Confirm Exit?"() -> (w1261:bool)
        n1038 = local read "Taking Data"() -> (w1260:bool)
        n1039 = Or(x=w1261, y=w1260) -> (x .or. y?=w1259:bool)
        n1040 = case shown="True" w1259 {
          tunnel: [TRUE ("T button?") w1265] -> w1263
          frame False {
          }
          frame True {
            n1041 = Two Button Dialog(message="Are you sure you would like to quit?", 1:"No" ("F button name (\"Cancel\")"), 2:"Yes" ("T button name (\"OK\")")) -> (T button?=w1265:bool)
          }
        }
        n1042 = case shown="True" w1263 {
          frame False {
          }
          frame True {
            n1043 = property class="App"() -> ("Application:Kind"=w1269:T13)  [unwired: 2 in, 2 out]
            n1044 = case shown="\"Development System\"" w1269 {
              frame "Development System" {
                n1045 = local write "Start/Stop"(FALSE) -> ()
                n1046 = local write "Close"(TRUE) -> ()
              }
              frame "Run Time System", Default {
                n1047 = Quit LabVIEW(quit? (T)=TRUE) -> ()
              }
            }
          }
        }
        n1048 = event-data("Discard?"=TRUE) -> ()  [unwired: 2 in, 1 out]
      }
      event Panel Close? {
        # "This event is duplicated in Application Exit?"
        n1049 = event-data() -> ()  [unwired: 1 in, 4 out]
        n1050 = local read "Confirm Exit?"() -> (w1275:bool)
        n1051 = local read "Taking Data"() -> (w1274:bool)
        n1052 = Or(x=w1275, y=w1274) -> (x .or. y?=w1273:bool)
        n1053 = case shown="True" w1273 {
          tunnel: [TRUE ("T button?") w1279] -> w1277
          frame False {
          }
          frame True {
            n1054 = Two Button Dialog(message="Are you sure you would like to quit?", 1:"No" ("F button name (\"Cancel\")"), 2:"Yes" ("T button name (\"OK\")")) -> (T button?=w1279:bool)
          }
        }
        n1055 = case shown="True" w1277 {
          frame False {
          }
          frame True {
            n1056 = property class="App"() -> ("Application:Kind"=w1283:T13)  [unwired: 2 in, 2 out]
            n1057 = case shown="\"Development System\"" w1283 {
              frame "Development System" {
                n1058 = local write "Start/Stop"(FALSE) -> ()
                n1059 = local write "Close"(TRUE) -> ()
              }
              frame "Run Time System", Default {
                n1060 = Quit LabVIEW(quit? (T)=TRUE) -> ()
              }
            }
          }
        }
        n1061 = event-data("Discard?"=TRUE) -> ()  [unwired: 1 in, 1 out]
      }
      event Timeout {
        n1062 = event-data() -> ()  [unwired: 1 in, 3 out]
      }
    }
  }
  "Confirm Exit?" <- FALSE
  "Version" <- "5.62" ("Version")
  "Voltage Overload" <- w1
  "Current Overload" <- w1
  "Control Amp Overload" <- w1
